vi "Anna_linescan2.0IngoHeucke.vi"() -> ()   [LabVIEW 2009]
panel:
  in  "Case Constant\n(See Context Help)":bool
  in  "Router":u32
  in  "save image to txt file":bool
  in  "threshold":cluster{"max":u32, "min":u32}
  in  "Header Path Ring":u16(ring)
  out "spots":i16
  in  "notes":string
  in  "new image":bool
  in  "exit":bool
  out "does a coinc image exist?":bool=TRUE
  in  "coincidence spot":bool
  in  "coincidence\nimage":bool
  out "LOADED HDR":bool
  out "Image LOADED":bool
  in  "settings":bool
  in  "Load Image":bool
  in  "F2-Image":bool
  in  "Lifetime pick":bool
  in  "Export":bool
  in  "TAC Window":bool
  in  "Spotfinder":bool
  in  "View FIFO Settings":bool
  in  "View Image Settings":bool
  in  "Load":bool
  out "total":i32
  out "gap":i32
  out "invalid":i32
  in  "plane":u32
  in  "router":u8(ring) items=["sum", "0", "1", "2", "3", "4", "5", "6"]
  in  "RGB or false color?":bool
  in  "16bit":bool
  out "already x spots":i16
  out "Int duplex?":bool
  out "16btimage?":bool
  out "Ampel":cluster{"RED":bool, "YELLOW":bool, "GREEN":bool}
  out "TACwinLoaded?":bool
  out "Boolean":bool
  in  "Image Path":path
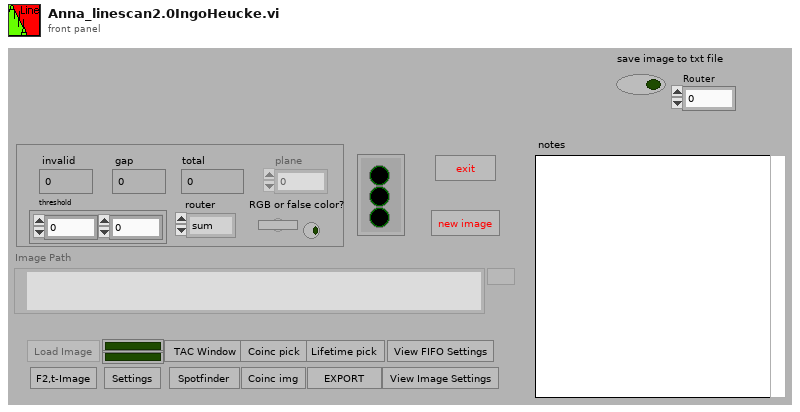
[diagram p1: front panel]
types:
  T1 = enum16{"Display", "change", "get", "save", "create text", "load", "Get Refnum"}
  T2 = enum16{"Get", "Set", "Change", "ini", "clear", "draw", "draw false"}
  T3 = enum16{"Ini", "Get", "Set", "Refresh", "dump", "move", "name"}
  T4 = enum16{"Ini", "Dump", "Colorpal", "Input", "Get"}
  T5 = enum16{"Display", "change", "Get", "Set", "Set Ken"}
  T6 = enum16{"Ini", "Get", "Set", "Draw", "Colorpal", "Dump", "Zoom"}
  T7 = cluster{"router":u8[], "macro times":dbl[], "micro times":u16[], "invalid":dbl[], "gap":dbl[]}
  T8 = typedef "Settings.ctl" = cluster{"threshold":cluster{"max":u32, "min":u32}, "RGB or false color":bool, "16bit":bool, "log/lin axis":u16, "spotsize button":bool, "Pixelsize":u16, "autoscale x":bool, "autoscale y":bool, "correlation":bool, "ADC-Resolution":i32, "F2-lifetime":cluster{"display tau":bool, "display F2":bool, "Palette Number lifetime":enum32{"Gray", "Binary", "Gradient", "Rainbow", "Temperature"}, "Palette Number F2":enum32{"Gray", "Binary", "Gradient", "Rainbow", "Temperature"}, "max tau-Value":dbl, "min tau-Value":dbl, "max F2-Value":dbl, "min F2-Value":dbl}, "TAC-Window 1":u16, "TAC-Window 2":u16, "false color palette":cluster{"1":u32, "2":u32, "3":u32, "4":u32, "5":u32, "6":u32, "7":u32, "8":u32, "8 2":u32, "8 3":u32, "8 4":u32, "8 5":u32}}
  T9 = enum32{"existing file", "new file", "new or existing file", "existing dir", "new dir", "new or existing dir", "existing file (use LLBs)", "new file (use LLBs)", "new or existing file (use LLBs)", "new or existing file or directory (use LLBs)"}
  T10 = typedef "ImageSettings.ctt" = cluster{"Start Position (µm)":cluster{"x":dbl, "y":dbl, "z":dbl}, "End Position (µm)":cluster{"x":dbl, "y":dbl, "z":dbl}, "Image Resolution (nm/pixel)":cluster{"x":dbl, "y":dbl, "z":dbl}, "Image Size (µm)":cluster{"x":dbl, "y":dbl, "z":dbl}, "Image Size (pixel)":cluster{"x":u32, "y":u32, "z":u32}, "Time Resolution\n(ms/pixel)":dbl, "1st Axis":u16, "2nd Axis":u16, "Retrace":bool, "Estimated Time":string}
  T11 = typedef "FIFOSettings_BH.ctt" = cluster{"Measurement":cluster{"Binning (ms)":sgl, "External Trigger Condition":u16, "Stop Condition:":u16, "Stop Count":dbl, "Buffer Size (Photons)":u16, "No of Channels":u16, "Ext Latch Delay":i16}, "ADC":cluster{"Module":u16, "ADC Resolution":i32, "Dither Range":i16, "Count Increment":i16, "Macro Time Clock":i16}, "SYNC":cluster{"SYNC ZC Level (mV)":sgl, "SYNC Freq Divider":i16, "SYNC Holdoff (ns)":sgl, "SYNC Threshold (mV)":sgl}, "TAC":cluster{"TAC Range (ns)":sgl, "TAC Gain":i16, "TAC Offset (%)":sgl, "TAC Limit Low (%)":sgl, "TAC Limit High (%)":sgl}, "CFD":cluster{"CFD Limit Low (mV)":sgl, "CFD Limit High (mV)":sgl, "CFD ZC Level (mV)":sgl, "CFD Holdoff (ns)":sgl}}
  T12 = typedef "spotproperties.ctl" = cluster{"draw?":bool, "plane":u32, "Coordinates":i32[], "TACWindow":cluster{"TACWindow1":i32, "TACWindow2":i32}, "Lifetime[ns]":ext[], "tauerror":dbl[], "F2-Value overall":dbl, "overall intensity":u32[], "F2-Value TAC":dbl, "TAC intensity":u32[], "Decay":u32[][]}
  T13 = enum16{"open", "replace", "create", "open or create", "replace or create", "replace or create with confirmation"}
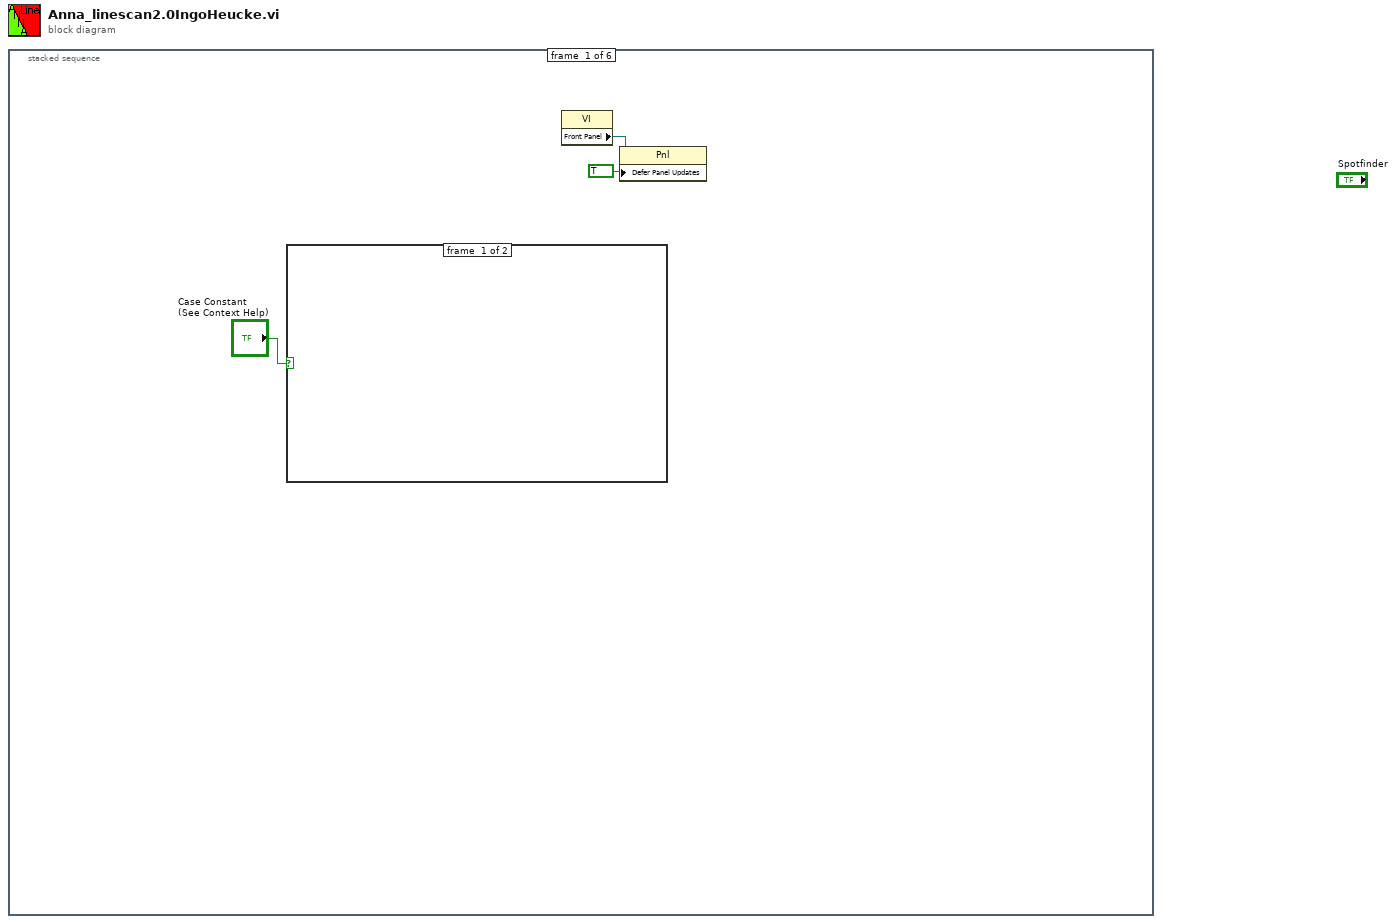
[diagram p0: block diagram]
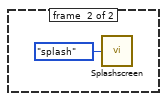
[diagram p2: hidden frame]
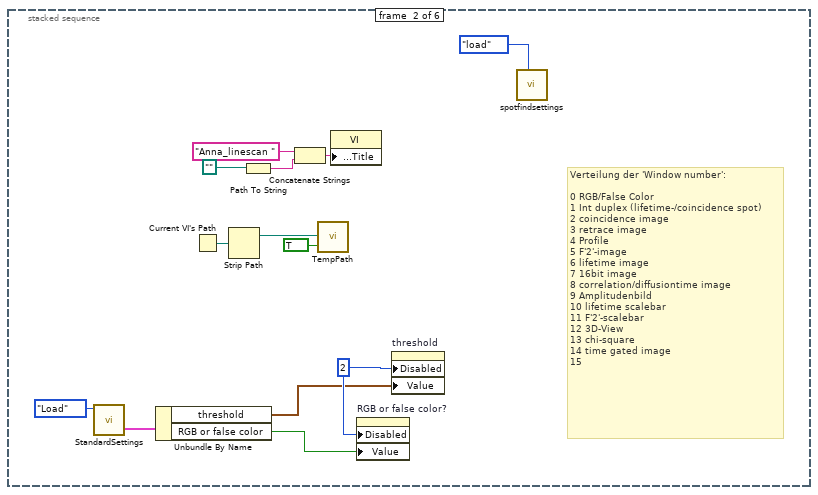
[diagram p3: hidden frame]
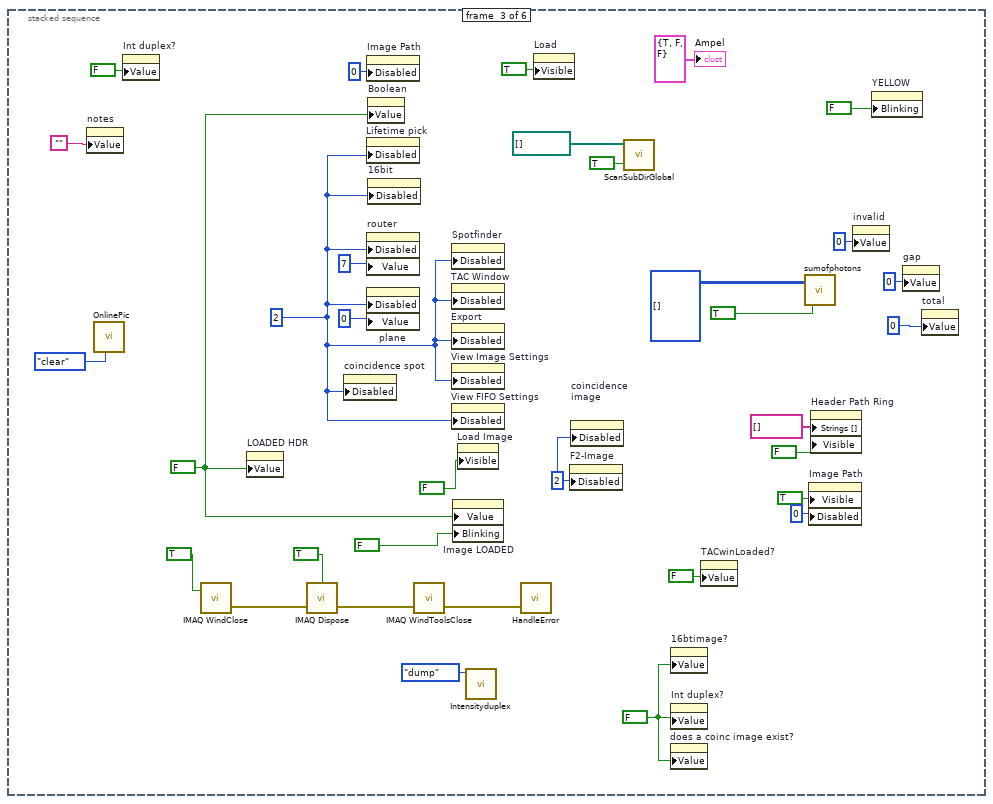
[diagram p4: hidden frame]
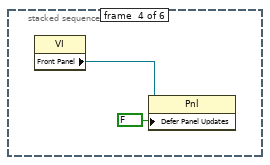
[diagram p5: hidden frame]
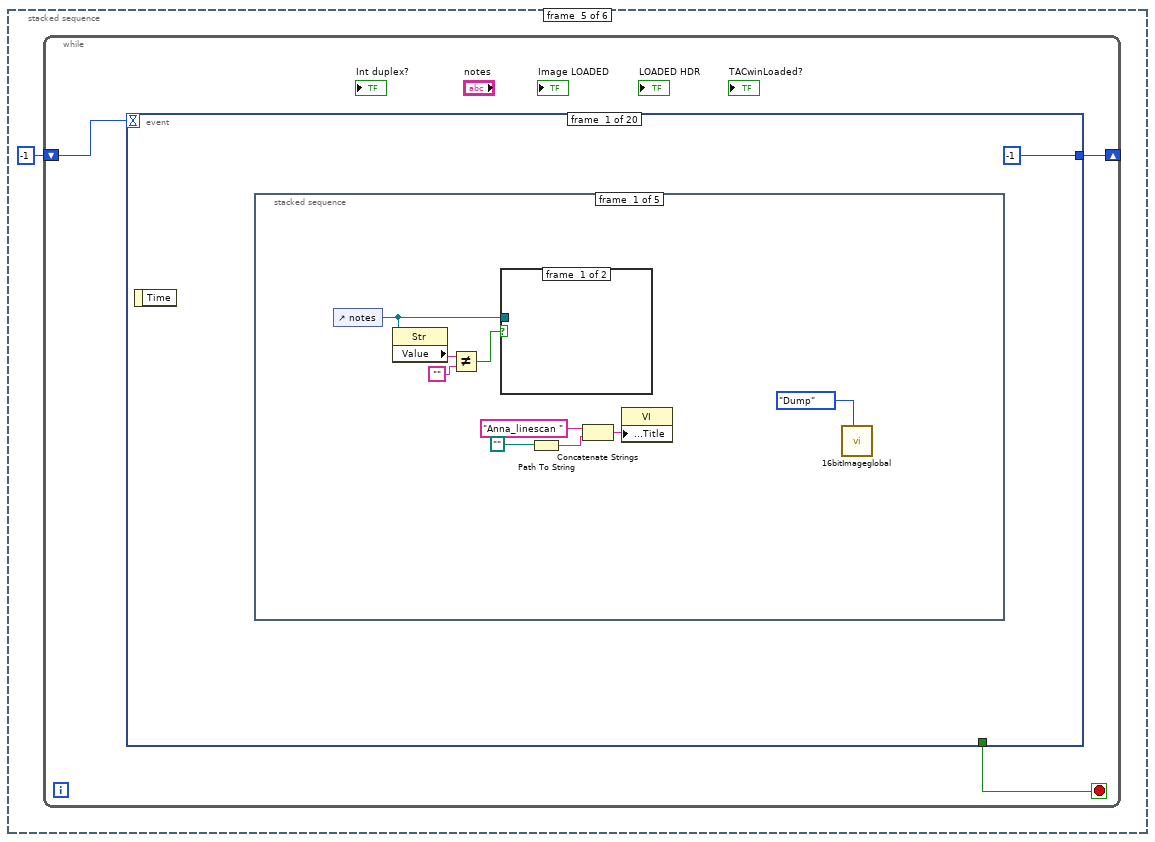
[diagram p6: hidden frame]
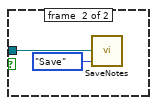
[diagram p7: hidden frame]
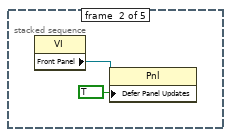
[diagram p8: hidden frame]
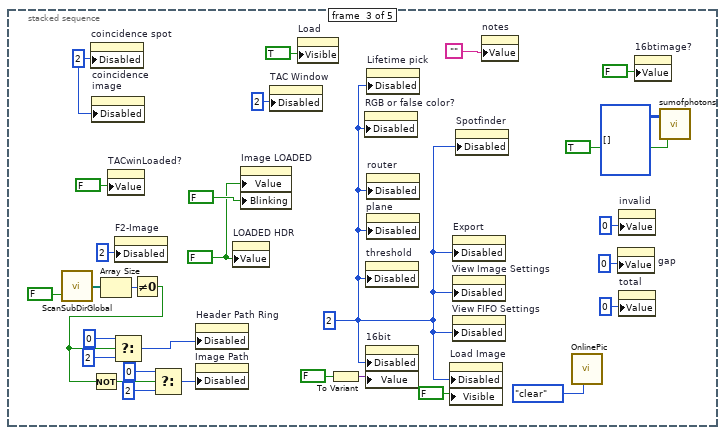
[diagram p9: hidden frame]
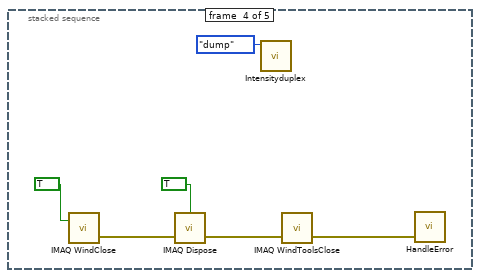
[diagram p10: hidden frame]
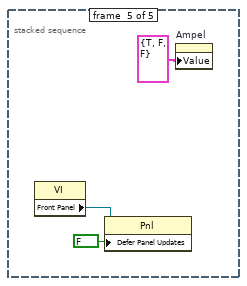
[diagram p11: hidden frame]
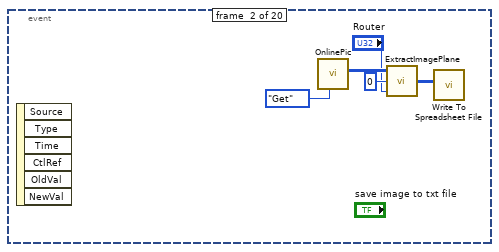
[diagram p12: hidden frame]
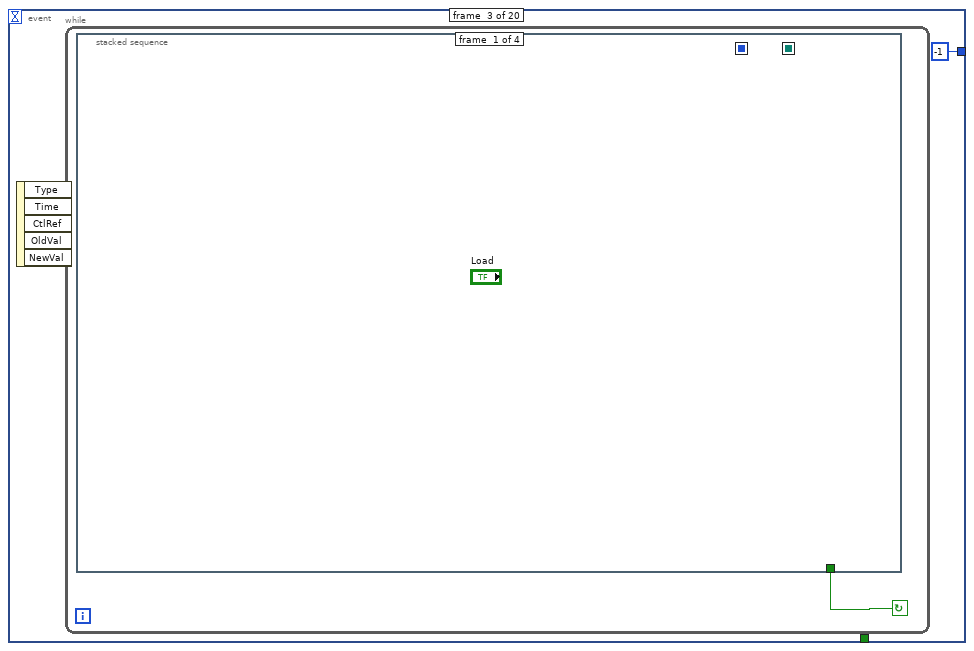
[diagram p13: hidden frame]
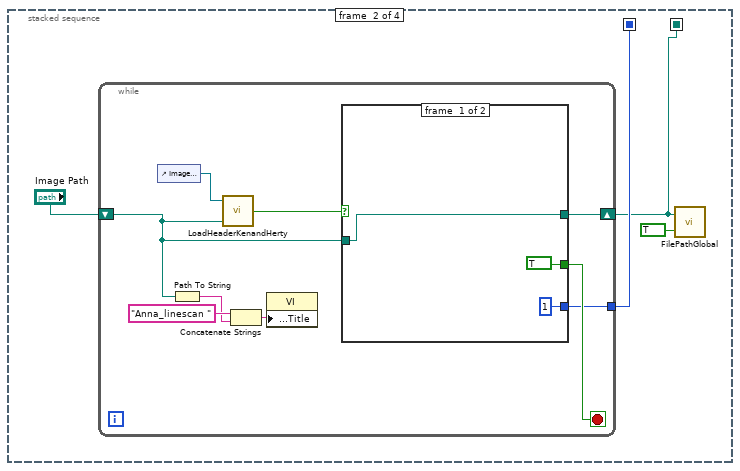
[diagram p14: hidden frame]
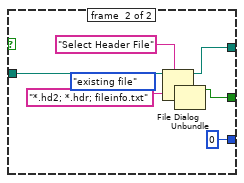
[diagram p15: hidden frame]
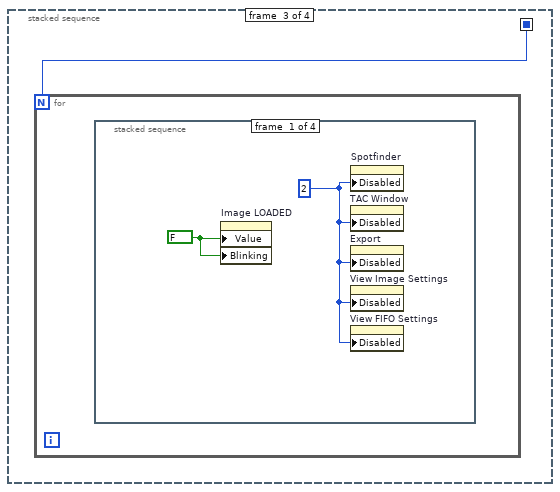
[diagram p16: hidden frame]
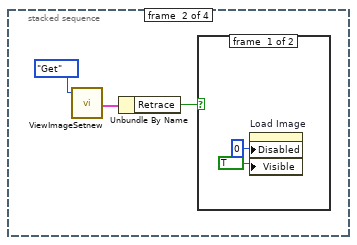
[diagram p17: hidden frame]
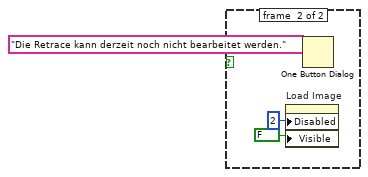
[diagram p18: hidden frame]
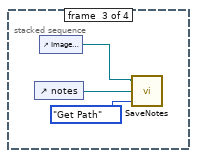
[diagram p19: hidden frame]
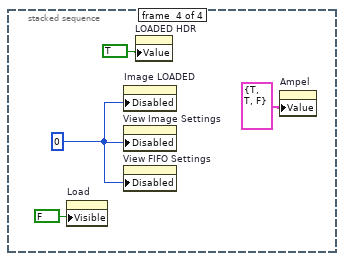
[diagram p20: hidden frame]
diagram:
  n1 = stacked-sequence {
    frame #0 {
      n2 = case shown="False" "Case Constant\n(See Context Help)" {
        frame #0 {
        }
        frame #1 {
          n3 = call "Splashscreen.vi"("Mode"=enum16{"splash", "dialog"}."splash") -> ()  [unwired: 1 in]
        }
      }
      n4 = property class="VI"() -> ("Front Panel"=w2:refnum<vi>)  [unwired: 2 in, 2 out]
      n5 = property class="Pnl"(reference=w2, "Defer Panel Updates"=TRUE) -> ()  [unwired: 1 in, 2 out]
    }
    frame #1 {
      w6 = u8 2 ("Disabled")
      # "Verteilung der 'Window number':\n\n0 RGB/False Color\n1 Int duplex (lifetime-/coincidence spot)\n2 coincidence image\n3 retrace image\n4 Profile\n5 F'2'-image\n6 lifetime image\n7 16bit image\n8 correlation/diffusiontime image\n9 Amplitudenbild\n10 lifetime scalebar\n11 F'2'-scalebar\n12 3D-View\n13 chi-square\n14 time gated image\n15"
      n6 = call "StandardSettings.vi"("Enum"=enum16{"Load", "get", "Save", "set"}."Load") -> ("StandardSettings"=w7:T8)  [unwired: 4 in]
      n7 = Unbundle By Name(w7) -> ("threshold"=w5:cluster{"max":u32, "min":u32}, "RGB or false color"=w8:bool)
      n8 = Current VI's Path() -> (path=w17:path)
      n9 = Strip Path(path=w17) -> (stripped path=w16:path)  [unwired: 1 out]
      n10 = Path To String(path=path "") -> (string=w12:string)
      n11 = Concatenate Strings("Anna_linescan " ("string"), w12) -> (w14:string)
      n12 = call "TempPath.vi"("change"=TRUE, "stripped path"=w16) -> ()  [unwired: 1 in, 1 out]
      n13 = property class="VI"("Front Panel Window:Title"=w14) -> ()  [unwired: 2 in, 2 out]
      n14 = property on="RGB or false color?" class="Boolean (strict)"("Disabled"=w6, "Value"=w8) -> ()  [unwired: 2 in, 2 out]
      n15 = property on="threshold" class="Clust (strict)"("Disabled"=w6, "Value"=w5) -> ()  [unwired: 2 in, 2 out]
      n16 = call "spotfindsettings.vi"("Enum"=T1."load") -> ()  [unwired: 8 in, 3 out]
    }
    frame #2 {
      w31 = FALSE
      w30 = u8 2 ("Disabled")
      w42 = FALSE ("Boolean")
      w20 = u8 2 ("Disabled")
      n17 = property on="notes" class="String"("Value"="") -> ()  [unwired: 2 in, 2 out]
      n18 = call "OnlinePic.vi"("action"=T2."clear" ("Enum")) -> ()  [unwired: 6 in, 5 out]
      n19 = property on="Int duplex?" class="Boolean (strict)"("Value"=FALSE ("Boolean 2")) -> ()  [unwired: 2 in, 2 out]
      n20 = call "IMAQ WindClose"("Close All Windows (False)"=TRUE ("Close All Windows (N)")) -> ("error out"=w47:errorcluster)  [unwired: 5 in]
      n21 = property on="LOADED HDR" class="Bool (strict)"("Value"=w42) -> ()  [unwired: 2 in, 2 out]
      n22 = call "IMAQ Dispose"("All Images? (No)"=TRUE, "error in (no error)"=w47) -> ("error out"=w48:errorcluster)  [unwired: 4 in]
      n23 = property on="coincidence spot" class="Boolean"("Disabled"=w20) -> ()  [unwired: 2 in, 2 out]
      n24 = property on="Image Path" class="Path"("Disabled"=u8 0) -> ()  [unwired: 2 in, 2 out]
      n25 = property on="Lifetime pick" class="Boolean"("Disabled"=w20) -> ()  [unwired: 2 in, 2 out]
      n26 = property on="router" class="Ring (strict)"("Disabled"=w20, "Value"=u8 7 ("router")) -> ()  [unwired: 2 in, 2 out]
      n27 = property on="plane" class="DigNum (strict)"("Disabled"=w20, "Value"=u32 0 ("plane")) -> ()  [unwired: 2 in, 2 out]
      n28 = property on="Boolean" class="Bool (strict)"("Value"=w42) -> ()  [unwired: 2 in, 2 out]
      n29 = property on="16bit" class="Boolean"("Disabled"=w20) -> ()  [unwired: 2 in, 2 out]
      n30 = call "IMAQ WindToolsClose"("error in (no error)"=w48) -> ("error out"=w46:errorcluster)  [unwired: 5 in]
      n31 = property on="Spotfinder" class="Boolean"("Disabled"=w20) -> ()  [unwired: 2 in, 2 out]
      n32 = property on="TAC Window" class="Boolean"("Disabled"=w20) -> ()  [unwired: 2 in, 2 out]
      n33 = property on="Export" class="Boolean"("Disabled"=w20) -> ()  [unwired: 2 in, 2 out]
      n34 = property on="View Image Settings" class="Boolean"("Disabled"=w20) -> ()  [unwired: 2 in, 2 out]
      n35 = property on="View FIFO Settings" class="Boolean"("Disabled"=w20) -> ()  [unwired: 2 in, 2 out]
      n36 = property on="Image LOADED" class="Boolean (strict)"("Value"=w42, "Blinking"=FALSE) -> ()  [unwired: 2 in, 2 out]
      n37 = property on="Load Image" class="Boolean"("Visible"=FALSE) -> ()  [unwired: 2 in, 2 out]
      n38 = call "Intensityduplex.vi"("Enum"=T3."dump") -> ()  [unwired: 4 in, 2 out]
      n39 = call "HandleError.vi"("error in (no error)"=w46) -> ()
      n40 = property on="Load" class="Bool"("Visible"=TRUE) -> ()  [unwired: 2 in, 2 out]
      n41 = property on="F2-Image" class="Boolean"("Disabled"=w30) -> ()  [unwired: 2 in, 2 out]
      n42 = property on="coincidence\nimage" class="Bool"("Disabled"=w30) -> ()  [unwired: 2 in, 2 out]
      n43 = call "ScanSubDirGlobal.vi"("set"=TRUE, "Array 2"=path[] []) -> ()  [unwired: 1 out]
      n44 = property on="16btimage?" class="Boolean (strict)"("Value"=w31) -> ()  [unwired: 2 in, 2 out]
      n45 = property on="Int duplex?" class="Boolean (strict)"("Value"=w31) -> ()  [unwired: 2 in, 2 out]
      n46 = property on="does a coinc image exist?" class="Boolean (strict)"("Value"=w31) -> ()  [unwired: 2 in, 2 out]
      n47 = property on="TACwinLoaded?" class="Boolean (strict)"("Value"=FALSE ("TACwinLoaded?")) -> ()  [unwired: 2 in, 2 out]
      n48 = call "sumofphotons.vi"("s"=TRUE, "sum of photons"=u32[][][][] []) -> ()  [unwired: 1 out]
      n49 = property on="Image Path" class="Path"("Visible"=TRUE, "Disabled"=u8 0) -> ()  [unwired: 2 in, 2 out]
      n50 = property on="Header Path Ring" class="Ring (strict)"("Strings []"=string[] [], "Visible"=FALSE) -> ()  [unwired: 2 in, 2 out]
      n51 = property on="invalid" class="DigNum (strict)"("Value"=u32 0 ("invalid photons")) -> ()  [unwired: 2 in, 2 out]
      n52 = property on="YELLOW" class="Boolean (strict)"("Blinking"=FALSE) -> ()  [unwired: 2 in, 2 out]
      n53 = property on="gap" class="DigNum (strict)"("Value"=u32 0 ("gap photons")) -> ()  [unwired: 2 in, 2 out]
      n54 = property on="total" class="DigNum (strict)"("Value"=u32 0 ("invalid photons")) -> ()  [unwired: 2 in, 2 out]
      "Ampel" <- cluster{"RED":bool, "YELLOW":bool, "GREEN":bool} {"RED"=TRUE, "YELLOW"=FALSE, "GREEN"=FALSE} ("Ampel")
    }
    frame #3 {
      n55 = property class="VI"() -> ("Front Panel"=w51:refnum<vi>)  [unwired: 2 in, 2 out]
      n56 = property class="Pnl"(reference=w51, "Defer Panel Updates"=FALSE) -> ()  [unwired: 1 in, 2 out]
    }
    frame #4 {
      n57 = while {
        shift-right: [w55] -> _
        shift-left: -1 -> [w54]
        stop <- w56 stop-if-true
        n58 = event shown="[2] \"Load\": Value Change" {
          selector: _ -> [_ _ _ _ _ _ _ _ _ _ _ _ _ _ _ _ _ _ _ _]
          dyn-events: _ -> [_ _ _ _ _ _ _ _ _ _ _ _ _ _ _ _ _ _ _ _]
          timeout: w54 -> [_ _ _ _ _ _ _ _ _ _ _ _ _ _ _ _ _ _ _ _]
          tunnel: [_ _ _ _ _ FALSE ("T button?") _ _ _ _ _ _ _ _ _ _ w463 _ TRUE w841] -> w56
          tunnel: [-1 _ -1 -1 -1 -1 100 -1 -1 -1 -1 -1 -1 -1 -1 -1 -1 -1 _ _] -> w55
          event #0 {
            n59 = event-data() -> ()  [unwired: 1 in, 1 out]
            n60 = stacked-sequence {
              frame #0 {
                n61 = control-ref of="notes"() -> (w66:refnum<vi>)
                n62 = property class="Str"(reference=w66) -> ("Value"=w59:string)  [unwired: 1 in, 2 out]
                n63 = Not Equal?(x=w59, y="") -> (x != y?=w58:bool)
                n64 = case shown="True" w58 {
                  tunnel: w66 -> [_ w67]
                  frame #0 {
                  }
                  frame #1 {
                    n65 = call "SaveNotes.vi"("Enum"=enum16{"Get Path", "Read", "Save"}."Save", "String"=w67) -> ()  [unwired: 3 in]
                  }
                }
                n66 = Path To String(path=path "") -> (string=w63:string)
                n67 = Concatenate Strings("Anna_linescan " ("string"), w63) -> (w65:string)
                n68 = property class="VI"("Front Panel Window:Title"=w65) -> ()  [unwired: 2 in, 2 out]
                n69 = call "16bitImageglobal.vi"("Enum"=T4."Dump") -> ()  [unwired: 4 in, 4 out]
              }
              frame #1 {
                n70 = property class="VI"() -> ("Front Panel"=w69:refnum<vi>)  [unwired: 2 in, 2 out]
                n71 = property class="Pnl"(reference=w69, "Defer Panel Updates"=TRUE) -> ()  [unwired: 1 in, 2 out]
              }
              frame #2 {
                w80 = u8 2 ("Disabled")
                w76 = FALSE ("Boolean")
                w71 = u8 2 ("Disabled")
                n72 = call "ScanSubDirGlobal.vi"("set"=FALSE) -> ("Array"=w89:path[])  [unwired: 1 in]
                n73 = property on="coincidence spot" class="Bool"("Disabled"=w80) -> ()  [unwired: 2 in, 2 out]
                n74 = property on="coincidence\nimage" class="Bool"("Disabled"=w80) -> ()  [unwired: 2 in, 2 out]
                n75 = Array Size(array=w89) -> (size(s)=w88:i32)
                n76 = property on="TACwinLoaded?" class="Boolean (strict)"("Value"=FALSE ("TACwinLoaded?")) -> ()  [unwired: 2 in, 2 out]
                n77 = property on="F2-Image" class="Boolean"("Disabled"=u8 2) -> ()  [unwired: 2 in, 2 out]
                n78 = Not Equal To 0?(x=w88) -> (x != 0?=w85:bool)
                n79 = Not(x=w85) -> (.not. x?=w84:bool)
                n80 = Select(t=u8 0 ("Disabled"), s=w85, f=u8 2 ("Disabled")) -> (s? t:f=w83:u8)
                n81 = Select(t=u8 0 ("Disabled"), s=w84, f=u8 2 ("Disabled")) -> (s? t:f=w82:u8)
                n82 = property on="Header Path Ring" class="Ring (strict)"("Disabled"=w83) -> ()  [unwired: 2 in, 2 out]
                n83 = property on="Image Path" class="Path"("Disabled"=w82) -> ()  [unwired: 2 in, 2 out]
                n84 = property on="LOADED HDR" class="Bool (strict)"("Value"=w76) -> ()  [unwired: 2 in, 2 out]
                n85 = property on="Image LOADED" class="Boolean (strict)"("Value"=w76, "Blinking"=FALSE) -> ()  [unwired: 2 in, 2 out]
                n86 = property on="TAC Window" class="Boolean"("Disabled"=2) -> ()  [unwired: 2 in, 2 out]
                n87 = property on="Load" class="Bool"("Visible"=TRUE) -> ()  [unwired: 2 in, 2 out]
                n88 = To Variant(anything=FALSE ("16btimage?")) -> (Variant=w73:variant)
                n89 = property on="RGB or false color?" class="Boolean (strict)"("Disabled"=w71) -> ()  [unwired: 2 in, 2 out]
                n90 = property on="threshold" class="Clust (strict)"("Disabled"=w71) -> ()  [unwired: 2 in, 2 out]
                n91 = property on="16bit" class="Boolean"("Disabled"=w71, "Value"=w73) -> ()  [unwired: 2 in, 2 out]
                n92 = property on="Lifetime pick" class="Boolean"("Disabled"=w71) -> ()  [unwired: 2 in, 2 out]
                n93 = property on="router" class="Ring (strict)"("Disabled"=w71) -> ()  [unwired: 2 in, 2 out]
                n94 = property on="plane" class="DigNum (strict)"("Disabled"=w71) -> ()  [unwired: 2 in, 2 out]
                n95 = property on="Load Image" class="Boolean"("Disabled"=w71, "Visible"=FALSE) -> ()  [unwired: 2 in, 2 out]
                n96 = property on="Export" class="Boolean"("Disabled"=w71) -> ()  [unwired: 2 in, 2 out]
                n97 = property on="View Image Settings" class="Boolean"("Disabled"=w71) -> ()  [unwired: 2 in, 2 out]
                n98 = property on="View FIFO Settings" class="Boolean"("Disabled"=w71) -> ()  [unwired: 2 in, 2 out]
                n99 = property on="Spotfinder" class="Boolean"("Disabled"=w71) -> ()  [unwired: 2 in, 2 out]
                n100 = property on="notes" class="String"("Value"="") -> ()  [unwired: 2 in, 2 out]
                n101 = call "OnlinePic.vi"("action"=T2."clear" ("Enum")) -> ()  [unwired: 6 in, 5 out]
                n102 = property on="gap" class="DigNum (strict)"("Value"=u32 0 ("gap photons")) -> ()  [unwired: 2 in, 2 out]
                n103 = property on="invalid" class="DigNum (strict)"("Value"=u32 0 ("invalid photons")) -> ()  [unwired: 2 in, 2 out]
                n104 = property on="total" class="DigNum (strict)"("Value"=u32 0 ("invalid photons")) -> ()  [unwired: 2 in, 2 out]
                n105 = property on="16btimage?" class="Boolean (strict)"("Value"=FALSE ("16btimage?")) -> ()  [unwired: 2 in, 2 out]
                n106 = call "sumofphotons.vi"("s"=TRUE, "sum of photons"=u32[][][][] []) -> ()  [unwired: 1 out]
              }
              frame #3 {
                n107 = call "IMAQ WindClose"("Close All Windows (False)"=TRUE ("Close All Windows (N)")) -> ("error out"=w104:errorcluster)  [unwired: 5 in]
                n108 = call "IMAQ Dispose"("All Images? (No)"=TRUE, "error in (no error)"=w104) -> ("error out"=w105:errorcluster)  [unwired: 4 in]
                n109 = call "Intensityduplex.vi"("Enum"=T3."dump") -> ()  [unwired: 4 in, 2 out]
                n110 = call "IMAQ WindToolsClose"("error in (no error)"=w105) -> ("error out"=w101:errorcluster)  [unwired: 5 in]
                n111 = call "HandleError.vi"("error in (no error)"=w101) -> ()
              }
              frame #4 {
                n112 = property class="VI"() -> ("Front Panel"=w107:refnum<vi>)  [unwired: 2 in, 2 out]
                n113 = property class="Pnl"(reference=w107, "Defer Panel Updates"=FALSE) -> ()  [unwired: 1 in, 2 out]
                n114 = property on="Ampel" class="Clust (strict)"("Value"=cluster{"RED":bool, "RED 2":bool, "RED 3":bool} {"RED"=TRUE, "RED 2"=FALSE, "RED 3"=FALSE} ("Ampel")) -> ()  [unwired: 2 in, 2 out]
              }
            }
          }
          event #1 {
            n115 = event-data() -> ()  [unwired: 1 in, 6 out]
            n116 = call "OnlinePic.vi"("action"=enum16{"Get", "Set", "Change", "ini"}."Get" ("Enum")) -> ("Sum of Photons"=w113:u32[][][][])  [unwired: 6 in, 4 out]
            n117 = call "ExtractImagePlane.vi"("Router"="Router", "Plane"=u32 0, "Trace"=w113) -> ("Intensity"=w110:u32[][])
            n118 = call "Write To Spreadsheet File.vi"("2D data"=w110) -> ()  [unwired: 7 in, 1 out]
          }
          event #2 {
            n119 = event-data() -> ()  [unwired: 1 in, 5 out]
            n120 = while {
              stop <- w116 continue-if-true
              n121 = stacked-sequence {
                seq-local: [_ w119 _ _] -> [_ _ w140 _]
                seq-local: [_ w117 _ _] -> [_ _ _ w159]
                tunnel: [_ _ _ w158] -> w116
                frame #0 {
                }
                frame #1 {
                  n122 = while {
                    shift-right: [w122] -> w117
                    shift-left: "Image Path" -> [w123]
                    tunnel: [w121] -> w119
                    stop <- w124 stop-if-true
                    n123 = control-ref of="Image Path"() -> (w129:refnum<vi>)
                    n124 = Path To String(path=w123) -> (string=w126:string)
                    n125 = call "LoadHeaderKenandHerty.vi"("appended path"=w123, "reference"=w129) -> ("unsuccesful?"=w125:bool)  [unwired: 3 in]
                    n126 = Concatenate Strings("Anna_linescan " ("string"), w126) -> (w128:string)
                    n127 = property class="VI"("Front Panel Window:Title"=w128) -> ()  [unwired: 2 in, 2 out]
                    n128 = case shown="False" w125 {
                      tunnel: w123 -> [w130 w139]
                      tunnel: [TRUE w135] -> w124
                      tunnel: [w130 w137] -> w122
                      tunnel: [1 0] -> w121
                      frame #0 {
                      }
                      frame #1 {
                        (unwired) T9."existing file" ("select mode (2)")
                        n129 = File Dialog(6:"*.hd2; *.hdr; fileinfo.txt" ("pattern"), 7:"Select Header File" ("prompt"), 11:w139) -> (0:w133:errorcluster, 1:w135:bool, 3:w137:path)  [unwired: 4 in, 1 out]
                        n130 = Unbundle(w133) -> ()  [unwired: 3 out]
                      }
                    }
                  }
                  n131 = call "FilePathGlobal.vi"("Image Path"=w117, "set?"=TRUE) -> ()  [unwired: 3 out]
                }
                frame #2 {
                  n132 = for {
                    N: w140 -> [_]
                    n133 = stacked-sequence {
                      frame #0 {
                        w142 = u8 2 ("Disabled")
                        w141 = FALSE ("Boolean")
                        n134 = property on="Image LOADED" class="Boolean (strict)"("Value"=w141, "Blinking"=w141) -> ()  [unwired: 2 in, 2 out]
                        n135 = property on="Spotfinder" class="Boolean"("Disabled"=w142) -> ()  [unwired: 2 in, 2 out]
                        n136 = property on="TAC Window" class="Boolean"("Disabled"=w142) -> ()  [unwired: 2 in, 2 out]
                        n137 = property on="Export" class="Boolean"("Disabled"=w142) -> ()  [unwired: 2 in, 2 out]
                        n138 = property on="View Image Settings" class="Boolean"("Disabled"=w142) -> ()  [unwired: 2 in, 2 out]
                        n139 = property on="View FIFO Settings" class="Boolean"("Disabled"=w142) -> ()  [unwired: 2 in, 2 out]
                      }
                      frame #1 {
                        n140 = call "ViewImageSetnew.vi"("action"=enum16{"Display", "change", "Get", "Set"}."Get" ("Enum")) -> ("Image Settings"=w144:T10)  [unwired: 2 in]
                        n141 = Unbundle By Name(w144) -> ("Retrace"=w143:bool)
                        n142 = case shown="False" w143 {
                          frame #0 {
                            n143 = property on="Load Image" class="Boolean"("Disabled"=u8 0, "Visible"=TRUE) -> ()  [unwired: 2 in, 2 out]
                          }
                          frame #1 {
                            n144 = property on="Load Image" class="Boolean"("Disabled"=u8 2, "Visible"=FALSE) -> ()  [unwired: 2 in, 2 out]
                            n145 = One Button Dialog(message="Die Retrace kann derzeit noch nicht bearbeitet werden.") -> ()  [unwired: 1 in, 1 out]
                          }
                        }
                      }
                      frame #2 {
                        n146 = control-ref of="notes"() -> (w153:refnum<vi>)
                        n147 = control-ref of="Image Path"() -> (w151:refnum<vi>)
                        n148 = call "SaveNotes.vi"("Enum"=enum16{"Get Path", "Read", "Save"}."Get Path", "String"=w153, "Path"=w151) -> ()  [unwired: 2 in]
                      }
                      frame #3 {
                        w156 = u8 0 ("Disabled")
                        n149 = property on="Load" class="Bool"("Visible"=FALSE) -> ()  [unwired: 2 in, 2 out]
                        n150 = property on="Image LOADED" class="Boolean (strict)"("Disabled"=w156) -> ()  [unwired: 2 in, 2 out]
                        n151 = property on="View Image Settings" class="Boolean"("Disabled"=w156) -> ()  [unwired: 2 in, 2 out]
                        n152 = property on="View FIFO Settings" class="Boolean"("Disabled"=w156) -> ()  [unwired: 2 in, 2 out]
                        n153 = property on="LOADED HDR" class="Bool (strict)"("Value"=TRUE ("Boolean")) -> ()  [unwired: 2 in, 2 out]
                        n154 = property on="Ampel" class="Clust (strict)"("Value"=cluster{"RED":bool, "RED 2":bool, "RED 3":bool} {"RED"=TRUE, "RED 2"=TRUE, "RED 3"=FALSE} ("Ampel")) -> ()  [unwired: 2 in, 2 out]
                      }
                    }
                  }
                }
                frame #3 {
                  n155 = stacked-sequence {
                    tunnel: [_ _ _ _ _ _ _ _ _ _ _ w241] -> _
                    tunnel: w159 -> [_ _ _ _ _ _ _ _ _ _ _ w241]
                    tunnel: [_ _ _ _ _ _ _ _ _ _ _ w228] -> w158
                    frame #0 {
                      n156 = property on="Image LOADED" class="Boolean (strict)"("Blinking"=TRUE) -> ()  [unwired: 2 in, 2 out]
                      n157 = property on="Image Path" class="Path"("Disabled"=u8 2) -> ()  [unwired: 2 in, 2 out]
                      n158 = property on="Load Image" class="Boolean"("Disabled"=u8 2) -> ()  [unwired: 2 in, 2 out]
                      n159 = call "sumofphotons.vi"("s"=TRUE, "sum of photons"=u32[][][][] []) -> ()  [unwired: 1 out]
                    }
                    frame #1 {
                      n160 = call "WriteTempData.vi"("Enum"=enum16{"create new", "write", "close"}."create new") -> ("error out"=w165:errorcluster)  [unwired: 4 in, 1 out]
                      n161 = call "HandleError.vi"("error in (no error)"=w165) -> ()
                    }
                    frame #2 {
                      n162 = call "fileformatGlobal.vi"("changed"=FALSE) -> ("fileformat out"=w167:enum16{"Herty", "Ken", "SPC130", "HydraHarp"})  [unwired: 1 in]
                      n163 = control-ref of="Image Path"() -> (w169:refnum<vi>)
                      n164 = case shown="\"HydraHarp\"" w167 {
                        tunnel: w169 -> [w170 w171 w172 w173]
                        frame #0 {
                          n165 = call "LoadData.vi"("Path"=w170) -> ()  [unwired: 2 in, 3 out]
                        }
                        frame #1 {
                          n166 = call "LoadDataSPC130.vi"("Path"=w171) -> ()  [unwired: 2 in, 3 out]
                        }
                        frame #2 {
                          n167 = call "LoadDataHH.vi"("Path"=w172) -> ()  [unwired: 2 in, 3 out]
                        }
                        frame #3 {
                          n168 = call "LoadDataKen.vi"("Path"=w173) -> ()  [unwired: 5 in]
                        }
                      }
                    }
                    frame #3 {
                      n169 = call "WriteTempData.vi"("Enum"=enum16{"create new", "write", "close"}."close") -> ("error out"=w174:errorcluster)  [unwired: 4 in, 1 out]
                      n170 = call "HandleError.vi"("error in (no error)"=w174) -> ()
                    }
                    frame #4 {
                      n171 = call "TotalRecall_Reload.vi"() -> ("gap"=→"gap":i32, "invalid"=→"invalid":i32, "valid"=→"total":i32)  [unwired: 4 in, 1 out]
                    }
                    frame #5 {
                      n172 = call "ViewFIFOSet.vi"("Enum"=T5."Get") -> ("FIFO Settings (Array)"=w185:T11[])  [unwired: 1 in]
                      n173 = Index Array(array=w185) -> (element=w186:T11)  [unwired: 1 in]
                      n174 = Array Size(array=w185) -> (size(s)=w181:i32)
                      n175 = Unbundle By Name(w186) -> ("Measurement.No of Channels"=w180:u16)
                      n176 = Multiply(x=w180, y=w181) -> (x*y=w179:i32)
                      n177 = for {
                        N: w179 -> [_]
                        tunnel: [w195] -> w184 mode=indexing
                        i -> [w196]
                        n178 = Number To Decimal String(number=w196) -> (decimal integer string=w195:string)  [unwired: 1 in]
                      }
                      n179 = Build Array (concatenate)("sum", w184) -> (w182:string[])
                      n180 = property on="router" class="Ring (strict)"("Strings []"=w182) -> ("Value"=w191:u8)  [unwired: 2 in, 2 out]
                      n181 = property on="plane" class="DigNum (strict)"() -> ("Value"=w192:u32)  [unwired: 2 in, 2 out]
                      n182 = property on="threshold" class="Clust (strict)"() -> ("Value"=w188:cluster{"max":u32, "min":u32})  [unwired: 2 in, 2 out]
                      n183 = call "sumofphotons.vi"("s"=FALSE) -> ("sum of photons out"=w189:u32[][][][])  [unwired: 1 in]
                      n184 = property on="RGB or false color?" class="Bool (strict)"() -> ("Value"=w193:bool)  [unwired: 2 in, 2 out]
                      n185 = call "OnlinePic.vi"("action"=T2."ini" ("Enum"), "RGB/False"=w193, "Threshold (max)"=w188, "plane"=w192, "router channel"=w191, "Array"=w189) -> ()  [unwired: 1 in, 5 out]
                    }
                    frame #6 {
                      n186 = call "ViewImageSetnew.vi"("action"=enum16{"Display", "change", "Get", "Set"}."Get" ("Enum")) -> ("Image Settings"=w198:T10)  [unwired: 2 in]
                      n187 = Unbundle By Name(w198) -> ("Image Size (pixel).z"=w199:u32)
                      n188 = case shown="0" w199 {
                        tunnel: [i8 2 w204] -> w200
                        tunnel: [u8 0 w204] -> w201
                        frame #0 {
                        }
                        frame #1 {
                          w204 = u8 0
                        }
                      }
                      n189 = property on="plane" class="DigNum (strict)"("Disabled"=w200, "Value"=w201) -> ()  [unwired: 2 in, 2 out]
                    }
                    frame #7 {
                      w205 = u8 0
                      n190 = property on="Image LOADED" class="Boolean (strict)"("Blinking"=FALSE, "Value"=TRUE ("Image LOADED")) -> ()  [unwired: 2 in, 2 out]
                      n191 = property on="Lifetime pick" class="Boolean"("Disabled"=w205) -> ()  [unwired: 2 in, 2 out]
                      n192 = property on="RGB or false color?" class="Boolean (strict)"("Disabled"=w205) -> ()  [unwired: 2 in, 2 out]
                      n193 = property on="16bit" class="Boolean"("Disabled"=w205) -> ()  [unwired: 2 in, 2 out]
                      n194 = property on="threshold" class="Clust (strict)"("Disabled"=w205) -> ()  [unwired: 2 in, 2 out]
                      n195 = property on="Spotfinder" class="Boolean"("Disabled"=w205) -> ()  [unwired: 2 in, 2 out]
                      n196 = property on="router" class="Ring (strict)"("Disabled"=w205) -> ()  [unwired: 2 in, 2 out]
                      n197 = property on="coincidence spot" class="Boolean"("Disabled"=w205) -> ()  [unwired: 2 in, 2 out]
                      n198 = property on="TAC Window" class="Boolean"("Disabled"=w205) -> ()  [unwired: 2 in, 2 out]
                      n199 = property on="Export" class="Bool"("Disabled"=w205) -> ()  [unwired: 2 in, 2 out]
                      n200 = property on="F2-Image" class="Boolean"("Disabled"=u8 0) -> ()  [unwired: 2 in, 2 out]
                      n201 = property on="coincidence\nimage" class="Bool"("Disabled"=w205) -> ()  [unwired: 2 in, 2 out]
                    }
                    frame #8 {
                      n202 = property on="Ampel" class="Clust (strict)"("Value"=cluster{"RED":bool, "RED 2":bool, "RED 3":bool} {"RED"=FALSE, "RED 2"=FALSE, "RED 3"=TRUE} ("Ampel")) -> ()  [unwired: 2 in, 2 out]
                    }
                    frame #9 {
                      n203 = stacked-sequence {
                        frame #0 {
                          n204 = property on="Ampel" class="Clust (strict)"("Value"=cluster{"RED":bool, "YELLOW":bool, "GREEN":bool} {"RED"=FALSE, "YELLOW"=FALSE, "GREEN"=FALSE} ("Ampel")) -> ("Controls[]"=w213:refnum<vi>[])  [unwired: 2 in, 2 out]
                          n205 = Index Array(array=w213, index=1) -> (element=w211:refnum<vi>)
                          n206 = property class="Ctl"(reference=w211, "Blinking"=TRUE) -> ()  [unwired: 1 in, 2 out]
                        }
                        frame #1 {
                          n207 = control-ref of="plane"() -> (w218:refnum<vi>)
                          n208 = control-ref of="TACwinLoaded?"() -> (w220:refnum<vi>)
                          n209 = control-ref of="16btimage?"() -> (w219:refnum<vi>)
                          n210 = control-ref of="router"() -> (w217:refnum<vi>)
                          n211 = control-ref of="Image Path"() -> (w221:refnum<vi>)
                          n212 = control-ref of="notes"() -> (w216:refnum<vi>)
                          n213 = control-ref of="Int duplex?"() -> (w222:refnum<vi>)
                          n214 = call "SpotFinderIngoHeucke.vi"("auto"=FALSE, "Int duplex?"=w222, "notes"=w216, "router 3"=w217, "plane 2"=w218, "Image Path"=w221, "16bit?"=w219, "TACwinLoaded?"=w220) -> ()  [unwired: 3 in]
                        }
                        frame #2 {
                          n215 = property on="Ampel" class="Clust (strict)"("Value"=cluster{"RED":bool, "YELLOW":bool, "GREEN":bool} {"RED"=FALSE, "YELLOW"=FALSE, "GREEN"=TRUE} ("Ampel")) -> ("Controls[]"=w226:refnum<vi>[])  [unwired: 2 in, 2 out]
                          n216 = Index Array(array=w226, index=1) -> (element=w224:refnum<vi>)
                          n217 = property class="Ctl"(reference=w224, "Blinking"=FALSE) -> ()  [unwired: 1 in, 2 out]
                        }
                      }
                    }
                    frame #10 {
                    }
                    frame #11 {
                      # "next file"
                      n218 = Strip Path(path=w241) -> (stripped path=w240:path, name=w237:string)
                      n219 = Strip Path(path=w240) -> (stripped path=w234:path, name=w236:string)
                      n220 = Scan From String(format string="%d", input string=w236) -> (output 1=w238:i32)  [unwired: 3 in, 3 out]
                      n221 = Increment(x=w238) -> (x+1=w235:i32)
                      n222 = Number To Decimal String(number=w235) -> (decimal integer string=w233:string)  [unwired: 1 in]
                      n223 = Search and Replace String(input string=w237, search string=w236, replace string=w233) -> (result string=w231:string)  [unwired: 5 in, 3 out]
                      n224 = Build Path(base path=w234, name or relative path=w233) -> (appended path=w232:path)
                      n225 = Build Path(base path=w232, name or relative path=w231) -> (appended path=w229:path)
                      n226 = call <vilib>:"Check if File or Folder Exists.vi"("path"=w229) -> ("file or folder exists?"=w228:bool)  [unwired: 8 in, 2 out]
                      n227 = call "FilePathGlobal.vi"("Image Path"=w229, "set?"=TRUE) -> ()  [unwired: 3 out]
                      n228 = local write "Image Path"(w229) -> ()
                    }
                  }
                }
              }
            }
          }
          event #3 {
            n229 = event-data() -> ()  [unwired: 1 in, 5 out]
          }
          event #4 {
            n230 = event-data() -> ()  [unwired: 1 in, 5 out]
            n231 = Unbundle By Name("threshold") -> ("max"=w248:u32, "min"=w247:u32)
            n232 = call "CheckPlane.vi"("plane 2"="plane") -> ("plane"=w249:u32)
            n233 = Max & Min(x=w248, y=w247) -> (max(x,y)=w246:u32, min(x,y)=w245:u32)
            n234 = Bundle By Name(cluster="threshold", "max"=w246, "min"=w245) -> (w243:cluster{"max":u32, "min":u32})
            n235 = property on="threshold" class="Cluster (strict)"("Value"=w243) -> ()  [unwired: 2 in, 2 out]
            n236 = property on="plane" class="DigNum (strict)"("Value"=w249) -> ()  [unwired: 2 in, 2 out]
            n237 = property on="16btimage?" class="Bool (strict)"() -> ("Value"=w258:bool)  [unwired: 2 in, 2 out]
            n238 = call "OnlinePic.vi"("action"=T2."Change" ("Enum"), "RGB/False"="RGB or false color?", "Threshold (max)"=w243, "plane"=w249, "router channel"="router") -> ()  [unwired: 2 in, 5 out]
            n239 = call "StandardSettings.vi"("Enum"=enum16{"Load", "get", "Save", "set"}."get") -> ("StandardSettings"=w254:T8)  [unwired: 4 in]
            n240 = Bundle By Name(cluster=w254, "threshold"=w243, "RGB or false color"="RGB or false color?") -> (w253:T8)
            n241 = case shown="True" w258 {
              tunnel: "router" -> [_ w263]
              tunnel: w249 -> [_ w262]
              frame #0 {
              }
              frame #1 {
                n242 = call "16bitImageglobal.vi"("Enum"=T4."Input", "plane"=w262, "router"=w263) -> ("error out"=w260:errorcluster)  [unwired: 2 in, 3 out]
                n243 = call "HandleError.vi"("error in (no error)"=w260) -> ()
              }
            }
            n244 = call "StandardSettings.vi"("StandardSettings"=w253, "Enum"=enum16{"Load", "get", "Save", "set"}."set") -> ()  [unwired: 3 in, 1 out]
          }
          event #5 {
            n245 = event-data() -> ()  [unwired: 1 in, 5 out]
            n246 = stacked-sequence {
              seq-local: [_ _ _ w294 _] -> [_ _ _ _ w299]
              frame #0 {
                n247 = property on="Ampel" class="Clust (strict)"("Value"=cluster{"RED":bool, "RED 2":bool, "RED 3":bool} {"RED"=FALSE, "RED 2"=FALSE, "RED 3"=FALSE} ("Ampel")) -> ()  [unwired: 2 in, 2 out]
                n248 = property on="TACwinLoaded?" class="Boolean (strict)"() -> ("Value"=w269:bool)  [unwired: 2 in, 2 out]
                n249 = call "Intensityduplex.vi"("Enum"=T3."dump") -> ()  [unwired: 4 in, 2 out]
                n250 = case shown="False" w269 {
                  frame #0 {
                    n251 = call "GetTACWindow.vi"("Enum"=enum16{"ini", "get", "quick"}."quick") -> ()  [unwired: 1 in, 9 out]
                  }
                  frame #1 {
                  }
                }
                n252 = property on="YELLOW" class="Boolean (strict)"("Blinking"=TRUE) -> ()  [unwired: 2 in, 2 out]
              }
              frame #1 {
                n253 = property on="threshold" class="Clust (strict)"() -> ("Value"=w271:cluster{"max":u32, "min":u32})  [unwired: 2 in, 2 out]
                n254 = call "StandardSettings.vi"("Enum"=enum16{"Load", "get", "Save", "set"}."get") -> ("StandardSettings"=w273:T8)  [unwired: 4 in]
                n255 = Bundle By Name(cluster=w273, "threshold"=w271) -> (w272:T8)
                n256 = property on="notes" class="String"() -> ("Value"=w277:string)  [unwired: 2 in, 2 out]
                n257 = Concatenate Strings(w277, "\n- lifetime picking" ("string")) -> (w276:string)
                n258 = call "StandardSettings.vi"("StandardSettings"=w272, "Enum"=enum16{"Load", "get", "Save", "set"}."set") -> ()  [unwired: 3 in, 1 out]
                n259 = control-ref of="Image Path"() -> (w281:refnum<vi>)
                n260 = property on="notes" class="String"("Value"=w276) -> ()  [unwired: 2 in, 2 out]
                n261 = call "WriteStoreData.vi"("Enum"=enum16{"Save", "Control"}."Control", "Image Path"=w281) -> ("already x spots"=→"already x spots":i16)  [unwired: 1 in]
              }
              frame #2 {
                n262 = property on="already x spots" class="Digital (strict)"() -> ("Value"=w284:i16)  [unwired: 2 in, 2 out]
                n263 = control-ref of="notes"() -> (w283:refnum<vi>)
                n264 = call "LifetimePickTACCube.vi"("notes 2"=w283, "already x spots"=w284) -> ("spots"=→"spots":i16)  [unwired: 1 in]
              }
              frame #3 {
                w293 = "%02d to %02d" ("format string")
                n265 = property on="already x spots" class="Digital (strict)"() -> ("Value"=w292:i16)  [unwired: 2 in, 2 out]
                n266 = property on="spots" class="Digital (strict)"() -> ("Value"=w291:i16)  [unwired: 2 in, 2 out]
                n267 = Greater?(x=w292, y=w291) -> (0:w290:bool)
                n268 = Decrement(x=w291) -> (x-1=w295:i16)
                n269 = Format Into String(format string=w293, initial string=" spots ", w292, w295) -> ()  [unwired: 1 in, 2 out]
                n270 = Format Into String(format string=w293, w292, w295) -> (resulting string=w294:string)  [unwired: 2 in, 1 out]
                n271 = Select(t=w293, s=w290, f="") -> (s? t:f=w288:string)
                n272 = call "Intensityduplex.vi"("Enum"=T3."name", "add string"=w288) -> ()  [unwired: 3 in, 2 out]
                n273 = call "OnlinePic.vi"("action"=T2."Get" ("Enum")) -> ("RGB/False out"=w286:bool, "Threshold (max) OUT"=w285:cluster{"max":u32, "min":u32})  [unwired: 6 in, 3 out]
                n274 = property on="RGB or false color?" class="Bool (strict)"("Value"=w286) -> ()  [unwired: 2 in, 2 out]
                n275 = property on="threshold" class="Clust (strict)"("Value"=w285) -> ()  [unwired: 2 in, 2 out]
              }
              frame #4 {
                n276 = call "StoreDatafromLifetimePick.vi"("Enum"=enum16{"clear", "Get", "Set", "Add"}."Get") -> ("Spots"=w298:T12[], "store s.th.?"=w303:bool)  [unwired: 1 in]
                n277 = case shown="True" w303 {
                  tunnel: w299 -> [_ w306]
                  tunnel: w298 -> [_ w305]
                  frame #0 {
                  }
                  frame #1 {
                    n278 = stacked-sequence {
                      tunnel: w306 -> [_ w311]
                      tunnel: w305 -> [w307 _]
                      frame #0 {
                        n279 = control-ref of="Image Path"() -> (w309:refnum<vi>)
                        n280 = call "WriteStoreData.vi"("Spots"=w307, "Enum"=enum16{"Save", "Control"}."Save", "Image Path"=w309) -> ()  [unwired: 1 out]
                      }
                      frame #1 {
                        n281 = property on="notes" class="String"() -> ("Value"=w313:string)  [unwired: 2 in, 2 out]
                        n282 = Concatenate Strings(w313, "\npick result spots (" ("string"), w311, ") and decays stored in IMAGE PATH\n" ("string")) -> (w312:string)
                        n283 = property on="notes" class="String"("Value"=w312) -> ()  [unwired: 2 in, 2 out]
                      }
                    }
                  }
                }
                n284 = property on="Int duplex?" class="Boolean (strict)"("Value"=TRUE ("Boolean 2")) -> ()  [unwired: 2 in, 2 out]
                n285 = property on="Ampel" class="Clust (strict)"("Value"=cluster{"RED":bool, "RED 2":bool, "RED 3":bool} {"RED"=FALSE, "RED 2"=FALSE, "RED 3"=TRUE} ("Ampel")) -> ()  [unwired: 2 in, 2 out]
                n286 = property on="YELLOW" class="Boolean (strict)"("Blinking"=FALSE) -> ()  [unwired: 2 in, 2 out]
              }
            }
          }
          event #6 {
            n287 = event-data() -> ()  [unwired: 1 in, 5 out]
          }
          event #7 {
            n288 = event-data() -> ()  [unwired: 1 in, 5 out]
            n289 = stacked-sequence {
              frame #0 {
              }
              frame #1 {
                n290 = control-ref of="Image Path"() -> (w317:refnum<vi>)
                n291 = call "GetSetTempDir.vi"("Path"=w317) -> ()  [unwired: 4 in]
              }
            }
          }
          event #8 {
            n292 = event-data() -> ()  [unwired: 1 in, 5 out]
            n293 = stacked-sequence {
              frame #0 {
                n294 = property on="Ampel" class="Clust (strict)"("Value"=cluster{"RED":bool, "RED 2":bool, "RED 3":bool} {"RED"=FALSE, "RED 2"=FALSE, "RED 3"=FALSE} ("Ampel")) -> ()  [unwired: 2 in, 2 out]
                n295 = property on="YELLOW" class="Boolean (strict)"("Blinking"=TRUE) -> ()  [unwired: 2 in, 2 out]
              }
              frame #1 {
                n296 = property on="Image LOADED" class="Bool (strict)"() -> ("Value"=w321:bool)  [unwired: 2 in, 2 out]
                n297 = case shown="True" w321 {
                  frame #0 {
                  }
                  frame #1 {
                    n298 = call "GetTACWindowIngoHeucke.vi"("Enum"=enum16{"ini", "get", "quick"}."ini") -> ("Cursor.Cursor Position:Cursor X"=w330:u16, "Cursor.Cursor Position:Cursor X 2"=w331:u16, "x-values"=w324:dbl[], "ready?"=w325:bool)  [unwired: 1 in, 5 out]
                    n299 = Select(t=2, s=w325, f=0) -> (s? t:f=w328:i32)
                    n300 = property on="TACwinLoaded?" class="Boolean (strict)"("Value"=TRUE ("TACwinLoaded?")) -> ()  [unwired: 2 in, 2 out]
                    n301 = call "CursorPositionChanged.vi"("CursorPos x1"=w331, "CursorPos x0"=w330, "x-values"=w324, "action"=enum16{"Check", "Get", "xval"}."xval" ("Enum")) -> ()  [unwired: 4 out]
                    n302 = property on="TAC Window" class="Boolean"("Disabled"=w328) -> ()  [unwired: 2 in, 2 out]
                  }
                }
              }
              frame #2 {
                n303 = property on="Ampel" class="Clust (strict)"("Value"=cluster{"RED":bool, "RED 2":bool, "RED 3":bool} {"RED"=FALSE, "RED 2"=FALSE, "RED 3"=TRUE} ("Ampel")) -> ()  [unwired: 2 in, 2 out]
                n304 = property on="YELLOW" class="Boolean (strict)"("Blinking"=FALSE) -> ()  [unwired: 2 in, 2 out]
                "Boolean" <- TRUE
              }
            }
          }
          event #9 {
            n305 = event-data() -> ()  [unwired: 1 in, 5 out]
          }
          event #10 {
            n306 = event-data() -> ()  [unwired: 1 in, 5 out]
            n307 = stacked-sequence {
              frame #0 {
              }
              frame #1 {
                n308 = control-ref of="Int duplex?"() -> (w341:refnum<vi>)
                n309 = control-ref of="16btimage?"() -> (w340:refnum<vi>)
                n310 = control-ref of="does a coinc image exist?"() -> (w339:refnum<vi>)
                n311 = control-ref of="Image Path"() -> (w338:refnum<vi>)
                n312 = control-ref of="notes"() -> (w337:refnum<vi>)
                n313 = call "ExportDialog.vi"("Int duplex ctl"=w341, "16 bit ctl"=w340, "coincidence image ctl"=w339, "Path"=w338, "notes 2"=w337) -> ()  [unwired: 4 in]
              }
            }
          }
          event #11 {
            n314 = event-data() -> ()  [unwired: 1 in, 5 out]
            n315 = stacked-sequence {
              frame #0 {
                n316 = property on="Ampel" class="Clust (strict)"("Value"=cluster{"RED":bool, "RED 2":bool, "RED 3":bool} {"RED"=FALSE, "RED 2"=FALSE, "RED 3"=FALSE} ("Ampel")) -> ()  [unwired: 2 in, 2 out]
                n317 = property on="YELLOW" class="Boolean (strict)"("Blinking"=TRUE) -> ()  [unwired: 2 in, 2 out]
              }
              frame #1 {
                n318 = property on="TACwinLoaded?" class="Bool (strict)"() -> ("Value"=w345:bool)  [unwired: 2 in, 2 out]
                n319 = case shown="False" w345 {
                  frame #0 {
                    n320 = call "GetTACWindowIngoHeucke.vi"("Enum"=enum16{"ini", "get", "quick"}."ini") -> ("Cursor.Cursor Position:Cursor X"=w349:u16, "Cursor.Cursor Position:Cursor X 2"=w348:u16, "x-values"=w347:dbl[])  [unwired: 1 in, 6 out]
                    n321 = call "CursorPositionChanged.vi"("CursorPos x1"=w348, "CursorPos x0"=w349, "x-values"=w347, "action"=enum16{"Check", "Get", "xval"}."xval" ("Enum")) -> ()  [unwired: 4 out]
                  }
                  frame #1 {
                  }
                }
              }
              frame #2 {
                n322 = property on="notes" class="String"() -> ("Value"=w352:string)  [unwired: 2 in, 2 out]
                n323 = Concatenate Strings(w352, "\n- F2 and lifetime image" ("string")) -> (w351:string)
                n324 = property on="notes" class="String"("Value"=w351) -> ()  [unwired: 2 in, 2 out]
              }
              frame #3 {
                n325 = property on="threshold" class="Clust (strict)"() -> ("Value"=w357:cluster{"max":u32, "min":u32})  [unwired: 2 in, 2 out]
                n326 = control-ref of="notes"() -> (w358:refnum<vi>)
                n327 = Unbundle(w357) -> ("max"=w356:u32, "min"=w355:u32)
                n328 = Max & Min(x=w356, y=w355) -> (min(x,y)=w354:u32)  [unwired: 1 out]
                n329 = control-ref of="Image Path"() -> (w359:refnum<vi>)
                n330 = call "ShowLifetimeAndF2Image.vi"("Path"=w359, "threshold (min)"=w354, "notes 2"=w358) -> ()  [unwired: 4 in]
              }
              frame #4 {
                n331 = property on="Ampel" class="Clust (strict)"("Value"=cluster{"RED":bool, "RED 2":bool, "RED 3":bool} {"RED"=FALSE, "RED 2"=FALSE, "RED 3"=TRUE} ("Ampel")) -> ()  [unwired: 2 in, 2 out]
                n332 = property on="YELLOW" class="Boolean (strict)"("Blinking"=FALSE) -> ()  [unwired: 2 in, 2 out]
              }
            }
          }
          event #12 {
            n333 = event-data() -> ()  [unwired: 1 in, 5 out]
            n334 = stacked-sequence {
              frame #0 {
                n335 = property on="16btimage?" class="Boolean (strict)"() -> ("Value"=w364:bool)  [unwired: 2 in, 2 out]
                n336 = Not(x=w364) -> (.not. x?=→"16btimage?":bool)
              }
              frame #1 {
                n337 = property on="16btimage?" class="Boolean (strict)"() -> ("Value"=w365:bool)  [unwired: 2 in, 2 out]
                n338 = case shown="True" w365 {
                  frame #0 {
                    n339 = call "16bitImageglobal.vi"("Enum"=T4."Dump") -> ()  [unwired: 4 in, 4 out]
                  }
                  frame #1 {
                    n340 = stacked-sequence {
                      frame #0 {
                        n341 = call "16bitImageglobal.vi"("Enum"=T4."Ini") -> ()  [unwired: 4 in, 4 out]
                      }
                      frame #1 {
                        n342 = property on="router" class="Ring (strict)"() -> ("Value"=w370:u8)  [unwired: 2 in, 2 out]
                        n343 = property on="plane" class="DigNum (strict)"() -> ("Value"=w369:u32)  [unwired: 2 in, 2 out]
                        n344 = call "16bitImageglobal.vi"("Enum"=T4."Input", "plane"=w369, "router"=w370) -> ()  [unwired: 2 in, 4 out]
                      }
                      frame #2 {
                        n345 = call "16bitImageglobal.vi"("Enum"=T4."Get") -> ()  [unwired: 4 in, 4 out]
                      }
                    }
                  }
                }
              }
            }
          }
          event #13 {
            n346 = event-data() -> ()  [unwired: 1 in, 5 out]
            n347 = stacked-sequence {
              frame #0 {
                n348 = property on="Ampel" class="Clust (strict)"("Value"=cluster{"RED":bool, "RED 2":bool, "RED 3":bool} {"RED"=FALSE, "RED 2"=FALSE, "RED 3"=FALSE} ("Ampel")) -> ()  [unwired: 2 in, 2 out]
                n349 = property on="YELLOW" class="Boolean (strict)"("Blinking"=TRUE) -> ()  [unwired: 2 in, 2 out]
                n350 = call "Intensityduplex.vi"("Enum"=T3."dump") -> ()  [unwired: 4 in, 2 out]
              }
              frame #1 {
                n351 = property on="notes" class="String"() -> ("Value"=w377:string)  [unwired: 2 in, 2 out]
                n352 = Concatenate Strings(w377, "\n- coincidence spotting" ("string")) -> (w376:string)
                n353 = property on="notes" class="String"("Value"=w376) -> ()  [unwired: 2 in, 2 out]
              }
              frame #2 {
                n354 = control-ref of="notes"() -> (w379:refnum<vi>)
                n355 = call "coincidenceImagenew.vi"("notes 2"=w379) -> ()  [unwired: 6 in]
              }
              frame #3 {
                n356 = property on="Ampel" class="Clust (strict)"("Value"=cluster{"RED":bool, "RED 2":bool, "RED 3":bool} {"RED"=FALSE, "RED 2"=FALSE, "RED 3"=TRUE} ("Ampel")) -> ()  [unwired: 2 in, 2 out]
                n357 = property on="YELLOW" class="Boolean (strict)"("Blinking"=FALSE) -> ()  [unwired: 2 in, 2 out]
              }
            }
          }
          event #14 {
            n358 = event-data() -> ()  [unwired: 1 in, 5 out]
            n359 = stacked-sequence {
              frame #0 {
                n360 = call "CoincidencePicture.vi"("Enum"=T6."Dump") -> ()  [unwired: 6 in, 3 out]
              }
              frame #1 {
                n361 = property on="notes" class="String"() -> ("Value"=w385:string)  [unwired: 2 in, 2 out]
                n362 = Concatenate Strings(w385, "\n- coincidence image" ("string")) -> (w384:string)
                n363 = property on="notes" class="String"("Value"=w384) -> ()  [unwired: 2 in, 2 out]
              }
              frame #2 {
                n364 = control-ref of="notes"() -> (w387:refnum<vi>)
                n365 = call "CoincidenceBuildImage.vi"("notes 2"=w387) -> ()  [unwired: 11 in]
              }
              frame #3 {
                n366 = call "CoincidencePicture.vi"("Enum"=enum16{"Ini", "Get", "Set", "Draw", "Colorpal"}."Get") -> ("String"=w390:string)  [unwired: 6 in, 2 out]
                n367 = Not Equal?(x=w390, y="") -> (x != y?=→"does a coinc image exist?":bool)
              }
            }
          }
          event #15 {
            n368 = event-data() -> ()  [unwired: 1 in, 5 out]
            n369 = stacked-sequence {
              frame #0 {
                n370 = call "ScanSubDirGlobal.vi"("set"=FALSE) -> ("Array"=w397:path[])  [unwired: 1 in]
                n371 = Index Array(array=w397, index="Header Path Ring") -> (element=w393:path)
                n372 = control-ref of="Image Path"() -> (w395:refnum<vi>)
                n373 = call "LoadHeaderKenandHerty.vi"("appended path"=w393, "reference"=w395) -> ("unsuccesful?"=w394:bool)  [unwired: 3 in]
                n374 = case shown="False" w394 {
                  tunnel: w393 -> [w399 _]
                  frame #0 {
                    n375 = call "FilePathGlobal.vi"("Image Path"=w399, "set?"=TRUE) -> ()  [unwired: 3 out]
                  }
                  frame #1 {
                  }
                }
              }
              frame #1 {
                n376 = control-ref of="notes"() -> (w401:refnum<vi>)
                n377 = control-ref of="Image Path"() -> (w403:refnum<vi>)
                n378 = call "SaveNotes.vi"("Enum"=enum16{"Get Path", "Read", "Save"}."Get Path", "String"=w401, "Path"=w403) -> ()  [unwired: 2 in]
              }
              frame #2 {
                w408 = u8 0 ("Disabled")
                n379 = property on="Load" class="Bool"("Visible"=FALSE) -> ()  [unwired: 2 in, 2 out]
                n380 = property on="Image LOADED" class="Boolean (strict)"("Disabled"=w408) -> ()  [unwired: 2 in, 2 out]
                n381 = property on="View Image Settings" class="Boolean"("Disabled"=w408) -> ()  [unwired: 2 in, 2 out]
                n382 = property on="View FIFO Settings" class="Boolean"("Disabled"=w408) -> ()  [unwired: 2 in, 2 out]
                n383 = property on="LOADED HDR" class="Bool (strict)"("Value"=TRUE ("Boolean")) -> ()  [unwired: 2 in, 2 out]
                n384 = property on="Ampel" class="Clust (strict)"("Value"=cluster{"RED":bool, "RED 2":bool, "RED 3":bool} {"RED"=TRUE, "RED 2"=TRUE, "RED 3"=FALSE} ("Ampel")) -> ()  [unwired: 2 in, 2 out]
                n385 = call "ViewImageSetnew.vi"("action"=enum16{"Display", "change", "Get", "Set"}."Get" ("Enum")) -> ("Image Settings"=w405:T10)  [unwired: 2 in]
                n386 = Unbundle By Name(w405) -> ("Retrace"=w406:bool)
                n387 = case shown="False" w406 {
                  frame #0 {
                    n388 = property on="Load Image" class="Boolean"("Disabled"=u8 0, "Visible"=TRUE) -> ()  [unwired: 2 in, 2 out]
                  }
                  frame #1 {
                    n389 = property on="Load Image" class="Boolean"("Disabled"=u8 2, "Visible"=FALSE) -> ()  [unwired: 2 in, 2 out]
                    n390 = One Button Dialog(message="Die Retrace kann derzeit noch nicht bearbeitet werden.") -> ()  [unwired: 1 in, 1 out]
                  }
                }
              }
              frame #3 {
                n391 = call "TempPath.vi"("change"=FALSE) -> ("stripped path 2"=w427:path)  [unwired: 2 in]
                n392 = Build Path(base path=w427, name or relative path="Anna_linescan.tmp" ("prompt")) -> (appended path=w425:path)
                n393 = property on="Image LOADED" class="Boolean (strict)"("Blinking"=TRUE) -> ()  [unwired: 2 in, 2 out]
                n394 = call <vilib>:"compatOverwrite.vi"("overwrite (F)"=TRUE) -> ("overwrite?"=w416:T13)
                n395 = Open/Create/Replace Datalog(5:T7 {"router"=[], "macro times"=[], "micro times"=[], "invalid"=[], "gap"=[]} ("cluster"), 10:w416, 11:w425) -> (3:w423:refnum<k1>)  [unwired: 3 in, 2 out]
                n396 = call "TempRefnum.vi"("change?"=TRUE, "refnum in"=w423) -> ()  [unwired: 1 out]
                n397 = property on="Header Path Ring" class="Ring (strict)"("Disabled"=u8 2) -> ()  [unwired: 2 in, 2 out]
                n398 = property on="Load Image" class="Boolean"("Disabled"=u8 2) -> ()  [unwired: 2 in, 2 out]
                n399 = call "sumofphotons.vi"("s"=TRUE, "sum of photons"=u32[][][][] []) -> ()  [unwired: 1 out]
              }
              frame #4 {
                n400 = control-ref of="Image Path"() -> (w430:refnum<vi>)
                n401 = call "fileformatGlobal.vi"("changed"=FALSE) -> ("fileformat out"=w432:enum16{"Herty", "Ken", "SPC130", "HydraHarp"})  [unwired: 1 in]
                n402 = case shown="\"Ken\"" w432 {
                  tunnel: w430 -> [w433 w434 w435]
                  frame #0 {
                    n403 = call "LoadData.vi"("Path"=w433) -> ()  [unwired: 2 in, 3 out]
                  }
                  frame #1 {
                    n404 = call "LoadDataSPC130.vi"("Path"=w434) -> ()  [unwired: 2 in, 3 out]
                  }
                  frame #2 {
                    n405 = call "LoadDataKen.vi"("Path"=w435) -> ()  [unwired: 5 in]
                  }
                }
              }
              frame #5 {
                n406 = stacked-sequence {
                  frame #0 {
                    n407 = call "TempRefnum.vi"("change?"=FALSE) -> ("refnum out"=w437:refnum<k1>)  [unwired: 1 in]
                    n408 = Close File(refnum=w437) -> (error out=w436:errorcluster)  [unwired: 1 in, 1 out]
                    n409 = call "HandleError.vi"("error in (no error)"=w436) -> ()
                  }
                  frame #1 {
                    n410 = call "TotalRecall_Reload.vi"() -> ("gap"=w439:i32, "invalid"=w440:i32, "valid"=w441:i32)  [unwired: 4 in, 1 out]
                    n411 = property on="total" class="DigNum (strict)"("Value"=w441) -> ()  [unwired: 2 in, 2 out]
                    n412 = property on="invalid" class="DigNum (strict)"("Value"=w440) -> ()  [unwired: 2 in, 2 out]
                    n413 = property on="gap" class="DigNum (strict)"("Value"=w439) -> ()  [unwired: 2 in, 2 out]
                  }
                  frame #2 {
                    n414 = call "sumofphotons.vi"("s"=FALSE) -> ("sum of photons out"=w443:u32[][][][])  [unwired: 1 in]
                    n415 = property on="plane" class="DigNum (strict)"() -> ("Value"=w446:u32)  [unwired: 2 in, 2 out]
                    n416 = property on="threshold" class="Clust (strict)"() -> ("Value"=w442:cluster{"max":u32, "min":u32})  [unwired: 2 in, 2 out]
                    n417 = property on="router" class="Ring (strict)"() -> ("Value"=w447:u8)  [unwired: 2 in, 2 out]
                    n418 = property on="RGB or false color?" class="Bool (strict)"() -> ("Value"=w448:bool)  [unwired: 2 in, 2 out]
                    n419 = call "OnlinePic.vi"("action"=T2."ini" ("Enum"), "RGB/False"=w448, "Threshold (max)"=w442, "plane"=w446, "router channel"=w447, "Array"=w443) -> ()  [unwired: 1 in, 5 out]
                  }
                  frame #3 {
                    n420 = call "ViewImageSetnew.vi"("action"=enum16{"Display", "change", "Get", "Set"}."Get" ("Enum")) -> ("Image Settings"=w452:T10)  [unwired: 2 in]
                    n421 = Unbundle By Name(w452) -> ("Image Size (pixel).z"=w451:u32)
                    n422 = case shown="0" w451 {
                      tunnel: [i8 2 w456] -> w450
                      tunnel: [u8 0 w456] -> w449
                      frame #0 {
                      }
                      frame #1 {
                        w456 = u8 0
                      }
                    }
                    n423 = property on="plane" class="DigNum (strict)"("Disabled"=w450, "Value"=w449) -> ()  [unwired: 2 in, 2 out]
                  }
                  frame #4 {
                    w457 = u8 0
                    n424 = property on="F2-Image" class="Boolean"("Disabled"=u8 0) -> ()  [unwired: 2 in, 2 out]
                    n425 = property on="Image LOADED" class="Boolean (strict)"("Blinking"=FALSE, "Value"=TRUE ("Image LOADED")) -> ()  [unwired: 2 in, 2 out]
                    n426 = property on="Lifetime pick" class="Boolean"("Disabled"=w457) -> ()  [unwired: 2 in, 2 out]
                    n427 = property on="RGB or false color?" class="Boolean (strict)"("Disabled"=w457) -> ()  [unwired: 2 in, 2 out]
                    n428 = property on="router" class="Ring (strict)"("Disabled"=w457) -> ()  [unwired: 2 in, 2 out]
                    n429 = property on="16bit" class="Boolean"("Disabled"=w457) -> ()  [unwired: 2 in, 2 out]
                    n430 = property on="threshold" class="Clust (strict)"("Disabled"=w457) -> ()  [unwired: 2 in, 2 out]
                    n431 = property on="coincidence spot" class="Boolean"("Disabled"=w457) -> ()  [unwired: 2 in, 2 out]
                    n432 = property on="TAC Window" class="Boolean"("Disabled"=w457) -> ()  [unwired: 2 in, 2 out]
                    n433 = property on="Export" class="Bool"("Disabled"=w457) -> ()  [unwired: 2 in, 2 out]
                    n434 = property on="coincidence\nimage" class="Bool"("Disabled"=w457) -> ()  [unwired: 2 in, 2 out]
                  }
                  frame #5 {
                    n435 = property on="Ampel" class="Clust (strict)"("Value"=cluster{"RED":bool, "RED 2":bool, "RED 3":bool} {"RED"=FALSE, "RED 2"=FALSE, "RED 3"=TRUE} ("Ampel")) -> ()  [unwired: 2 in, 2 out]
                  }
                }
              }
            }
          }
          event #16 {
            n436 = event-data() -> ("ItemTag"=w464:string)  [unwired: 1 in, 5 out]
            n437 = case shown="\"Spotfinder\"" w464 {
              tunnel: [_ _ TRUE _ _ _ _ _ _ _ _ _ _ _ _ _ _ _ _ _ _] -> w463
              frame #0 {
                n438 = control-ref of="Image Path"() -> (w465:refnum<vi>)
                n439 = property class="Path"(reference=w465) -> ("Value"=w466:path)  [unwired: 1 in, 2 out]
                n440 = Strip Path(path=w466) -> (stripped path=w467:path)  [unwired: 1 out]
                n441 = Not A Number/Path/Refnum?(number/path/refnum=w467) -> (NaN/Path/Refnum?=w468:bool)
                n442 = case shown="False" w468 {
                  tunnel: w467 -> [w471 _]
                  frame #0 {
                    n443 = call "fileformatGlobal.vi"() -> ("fileformat out"=w473:enum16{"Herty", "Ken", "SPC130", "HydraHarp"})  [unwired: 2 in]
                    n444 = case shown="\"SPC130\"" w473 {
                      tunnel: ["plane000line000.fifo" ("name or relative path") "plane000line000module000.spc" ("name or relative path") "0_0.ifif" ("name or relative path")] -> w472
                      frame #0 {
                      }
                      frame #1 {
                      }
                      frame #2 {
                      }
                    }
                    n445 = call "ViewFIFOSet.vi"("Enum"=enum16{"Display", "change", "Get", "Set"}."Get") -> ("FIFO Settings (Array)"=w479:T11[])  [unwired: 1 in]
                    n446 = Index Array(array=w479) -> (element=w469:T11)  [unwired: 1 in]
                    n447 = Unbundle By Name(w469) -> ("ADC.ADC Resolution"=w475:i32)
                    n448 = Not Equal To 0?(x=w475) -> (x != 0?=w474:bool)
                    n449 = Build Path(base path=w471, name or relative path=w472) -> (appended path=w470:path)
                    n450 = Select(t=enum16{"32 bit", "48 bit"}."48 bit" ("File Type"), s=w474, f=enum16{"32 bit", "48 bit"}."32 bit" ("File Type")) -> (s? t:f=w478:enum16{"32 bit", "48 bit"})
                    n451 = call "FIFORawDataScreener.vi"("File Type"=w478, "Path"=w470) -> ()  [unwired: 2 in]
                  }
                  frame #1 {
                    n452 = One Button Dialog(message="Select header file first!") -> ()  [unwired: 1 in, 1 out]
                  }
                }
              }
              frame #1 {
                n453 = call "ViewFIFOTrace.vi"() -> ()  [unwired: 1 in]
              }
              frame #2 {
              }
              frame #3 {
                n454 = stacked-sequence {
                  seq-local: [_ _ _ _ w519 _] -> [_ _ _ _ _ w531]
                  frame #0 {
                    n455 = control-ref of="notes"() -> (w490:refnum<vi>)
                    n456 = property class="Str"(reference=w490) -> (reference out=w486:refnum<vi>, "Value"=w488:string)  [unwired: 1 in, 1 out]
                    n457 = Not Equal?(x=w488, y="") -> (x != y?=w487:bool)
                    n458 = case shown="True" w487 {
                      tunnel: w486 -> [_ w491]
                      frame #0 {
                      }
                      frame #1 {
                        n459 = call "SaveNotes.vi"("Enum"=enum16{"Get Path", "Read", "Save"}."Save", "String"=w491) -> ()  [unwired: 3 in]
                      }
                    }
                  }
                  frame #1 {
                    w507 = FALSE ("Boolean")
                    w500 = u8 2 ("Disabled")
                    n460 = property on="TACwinLoaded?" class="Boolean (strict)"("Value"=FALSE ("TACwinLoaded?")) -> ()  [unwired: 2 in, 2 out]
                    n461 = property on="F2-Image" class="Boolean"("Disabled"=u8 2) -> ()  [unwired: 2 in, 2 out]
                    n462 = property on="TAC Window" class="Boolean"("Disabled"=2) -> ()  [unwired: 2 in, 2 out]
                    n463 = property on="LOADED HDR" class="Bool (strict)"("Value"=w507) -> ()  [unwired: 2 in, 2 out]
                    n464 = property on="Image LOADED" class="Boolean (strict)"("Value"=w507, "Blinking"=FALSE) -> ()  [unwired: 2 in, 2 out]
                    n465 = property on="Image Path" class="Path"("Disabled"=u8 0) -> ()  [unwired: 2 in, 2 out]
                    n466 = property on="Load" class="Bool"("Visible"=TRUE) -> ()  [unwired: 2 in, 2 out]
                    n467 = property on="RGB or false color?" class="Boolean (strict)"("Disabled"=w500, "Value"=w507) -> ()  [unwired: 2 in, 2 out]
                    n468 = property on="Lifetime pick" class="Boolean"("Disabled"=w500) -> ()  [unwired: 2 in, 2 out]
                    n469 = property on="router" class="Ring (strict)"("Disabled"=w500) -> ()  [unwired: 2 in, 2 out]
                    n470 = property on="plane" class="DigNum (strict)"("Disabled"=w500) -> ()  [unwired: 2 in, 2 out]
                    n471 = property on="Export" class="Boolean"("Disabled"=w500) -> ()  [unwired: 2 in, 2 out]
                    n472 = property on="View Image Settings" class="Boolean"("Disabled"=w500) -> ()  [unwired: 2 in, 2 out]
                    n473 = property on="View FIFO Settings" class="Boolean"("Disabled"=w500) -> ()  [unwired: 2 in, 2 out]
                    n474 = property on="Load Image" class="Boolean"("Disabled"=w500, "Visible"=FALSE) -> ()  [unwired: 2 in, 2 out]
                    n475 = property on="16bit" class="Boolean"("Disabled"=w500) -> ()  [unwired: 2 in, 2 out]
                    n476 = property on="Spotfinder" class="Boolean"("Disabled"=w500) -> ()  [unwired: 2 in, 2 out]
                    n477 = property on="notes" class="String"("Value"="") -> ()  [unwired: 2 in, 2 out]
                    n478 = property on="invalid" class="DigNum (strict)"("Value"=u32 0 ("invalid photons")) -> ()  [unwired: 2 in, 2 out]
                    n479 = property on="gap" class="DigNum (strict)"("Value"=u32 0 ("gap photons")) -> ()  [unwired: 2 in, 2 out]
                    n480 = property on="total" class="DigNum (strict)"("Value"=u32 0 ("invalid photons")) -> ()  [unwired: 2 in, 2 out]
                    n481 = call "sumofphotons.vi"("s"=TRUE, "sum of photons"=u32[][][][] []) -> ()  [unwired: 1 out]
                  }
                  frame #2 {
                    n482 = call "IMAQ WindClose"("Close All Windows (False)"=TRUE ("Close All Windows (N)")) -> ("error out"=w514:errorcluster)  [unwired: 5 in]
                    n483 = call "IMAQ Dispose"("All Images? (No)"=TRUE, "error in (no error)"=w514) -> ("error out"=w515:errorcluster)  [unwired: 4 in]
                    n484 = call "IMAQ WindToolsClose"("error in (no error)"=w515) -> ("error out"=w508:errorcluster)  [unwired: 5 in]
                    n485 = call "Intensityduplex.vi"("Enum"=T3."dump") -> ()  [unwired: 4 in, 2 out]
                    n486 = call "OnlinePic.vi"("action"=T2."clear" ("Enum")) -> ()  [unwired: 6 in, 5 out]
                    n487 = call "16bitImageglobal.vi"("Enum"=T4."Ini") -> ()  [unwired: 4 in, 4 out]
                    n488 = call "HandleError.vi"("error in (no error)"=w508) -> ()
                    n489 = Wait Until Next ms Multiple(millisecond multiple=u32 2500) -> ()  [unwired: 1 out]
                  }
                  frame #3 {
                    n490 = property on="Ampel" class="Clust (strict)"("Value"=cluster{"RED":bool, "RED 2":bool, "RED 3":bool} {"RED"=TRUE, "RED 2"=FALSE, "RED 3"=FALSE} ("Ampel")) -> ()  [unwired: 2 in, 2 out]
                  }
                  frame #4 {
                    (unwired) T9."existing file" ("select mode (2)")
                    n491 = File Dialog(6:"*.hdr; fileinfo.txt" ("pattern"), 7:"Select header file ... (quick view)" ("prompt")) -> (0:w518:errorcluster, 1:w520:bool, 3:w521:path)  [unwired: 5 in, 1 out]
                    n492 = Unbundle(w518) -> ()  [unwired: 3 out]
                    n493 = case shown="False" w520 {
                      tunnel: w521 -> [w526 _]
                      tunnel: [1 0] -> w519
                      frame #0 {
                        n494 = control-ref of="Image Path"() -> (w525:refnum<vi>)
                        n495 = call "LoadHeaderKenandHerty.vi"("appended path"=w526, "reference"=w525) -> ()  [unwired: 3 in, 1 out]
                        n496 = Path To String(path=w526) -> (string=w527:string)
                        n497 = Concatenate Strings("Anna_linescan " ("string"), w527) -> (w529:string)
                        n498 = property class="VI"("Front Panel Window:Title"=w529) -> ()  [unwired: 2 in, 2 out]
                      }
                      frame #1 {
                      }
                    }
                  }
                  frame #5 {
                    n499 = for {
                      N: w531 -> [_]
                      n500 = stacked-sequence {
                        frame #0 {
                          w532 = u8 0 ("Disabled")
                          n501 = property on="LOADED HDR" class="Bool (strict)"("Value"=TRUE ("Boolean")) -> ()  [unwired: 2 in, 2 out]
                          n502 = property on="Load" class="Bool"("Visible"=FALSE) -> ()  [unwired: 2 in, 2 out]
                          n503 = property on="Image LOADED" class="Boolean (strict)"("Disabled"=w532) -> ()  [unwired: 2 in, 2 out]
                          n504 = property on="View Image Settings" class="Boolean"("Disabled"=w532) -> ()  [unwired: 2 in, 2 out]
                          n505 = property on="View FIFO Settings" class="Boolean"("Disabled"=w532) -> ()  [unwired: 2 in, 2 out]
                          n506 = control-ref of="notes"() -> (w538:refnum<vi>)
                          n507 = control-ref of="Image Path"() -> (w536:refnum<vi>)
                          n508 = property on="Ampel" class="Clust (strict)"("Value"=cluster{"RED":bool, "RED 2":bool, "RED 3":bool} {"RED"=TRUE, "RED 2"=TRUE, "RED 3"=FALSE} ("Ampel")) -> ()  [unwired: 2 in, 2 out]
                          n509 = call "SaveNotes.vi"("Enum"=enum16{"Get Path", "Read", "Save"}."Get Path", "String"=w538, "Path"=w536) -> ()  [unwired: 2 in]
                        }
                        frame #1 {
                          n510 = call "ViewImageSetnew.vi"("action"=enum16{"Display", "change", "Get", "Set"}."Get" ("Enum")) -> ("Image Settings"=w540:T10)  [unwired: 2 in]
                          n511 = Unbundle By Name(w540) -> ("Retrace"=w539:bool)
                          n512 = case shown="False" w539 {
                            frame #0 {
                              n513 = property on="Load Image" class="Boolean"("Disabled"=u8 0, "Visible"=TRUE) -> ()  [unwired: 2 in, 2 out]
                            }
                            frame #1 {
                              n514 = property on="Load Image" class="Boolean"("Disabled"=u8 2, "Visible"=FALSE) -> ()  [unwired: 2 in, 2 out]
                              n515 = One Button Dialog(message="Die Retrace kann derzeit noch nicht bearbeitet werden.") -> ()  [unwired: 1 in, 1 out]
                            }
                          }
                        }
                        frame #2 {
                          n516 = property on="Image Path" class="Path"("Disabled"=u8 2) -> ()  [unwired: 2 in, 2 out]
                          n517 = property on="Load Image" class="Boolean"("Disabled"=u8 2) -> ()  [unwired: 2 in, 2 out]
                          n518 = property on="Image LOADED" class="Boolean (strict)"("Blinking"=TRUE) -> ()  [unwired: 2 in, 2 out]
                          n519 = call "sumofphotons.vi"("s"=TRUE, "sum of photons"=u32[][][][] []) -> ()  [unwired: 1 out]
                        }
                        frame #3 {
                          n520 = control-ref of="Image Path"() -> (w556:refnum<vi>)
                          n521 = call "fileformatGlobal.vi"() -> ("fileformat out"=w555:enum16{"Herty", "Ken", "SPC130", "HydraHarp"})  [unwired: 2 in]
                          n522 = call "QuickLoadData.vi"("Fileformat"=w555, "Path"=w556) -> ("gap photons"=w552:u32, "invalid photons"=w554:u32, "total"=w553:u32)  [unwired: 1 in]
                          n523 = property on="invalid" class="DigNum (strict)"("Value"=w553) -> ()  [unwired: 2 in, 2 out]
                          n524 = property on="total" class="DigNum (strict)"("Value"=w554) -> ()  [unwired: 2 in, 2 out]
                          n525 = property on="gap" class="DigNum (strict)"("Value"=w552) -> ()  [unwired: 2 in, 2 out]
                        }
                        frame #4 {
                          n526 = call "sumofphotons.vi"("s"=FALSE) -> ("sum of photons out"=w559:u32[][][][])  [unwired: 1 in]
                          n527 = property on="threshold" class="Clust (strict)"() -> ("Value"=w557:cluster{"max":u32, "min":u32})  [unwired: 2 in, 2 out]
                          n528 = property on="router" class="Ring (strict)"() -> ("Value"=w562:u8)  [unwired: 2 in, 2 out]
                          n529 = property on="plane" class="DigNum (strict)"() -> ("Value"=w563:u32)  [unwired: 2 in, 2 out]
                          n530 = property on="RGB or false color?" class="Bool (strict)"() -> ("Value"=w561:bool)  [unwired: 2 in, 2 out]
                          n531 = call "OnlinePic.vi"("action"=T2."ini" ("Enum"), "RGB/False"=w561, "Threshold (max)"=w557, "plane"=w563, "router channel"=w562, "Array"=w559) -> ()  [unwired: 1 in, 5 out]
                        }
                        frame #5 {
                          n532 = call "ViewImageSetnew.vi"("action"=enum16{"Display", "change", "Get", "Set"}."Get" ("Enum")) -> ("Image Settings"=w565:T10)  [unwired: 2 in]
                          n533 = Unbundle By Name(w565) -> ("Image Size (pixel).z"=w566:u32)
                          n534 = case shown="0" w566 {
                            tunnel: [i8 2 w571] -> w567
                            tunnel: [u8 0 w571] -> w568
                            frame #0 {
                            }
                            frame #1 {
                              w571 = u8 0
                            }
                          }
                          n535 = property on="plane" class="DigNum (strict)"("Disabled"=w567, "Value"=w568) -> ()  [unwired: 2 in, 2 out]
                        }
                        frame #6 {
                          w572 = u8 0
                          w573 = u8 2 ("Disabled")
                          n536 = property on="Image LOADED" class="Boolean (strict)"("Blinking"=FALSE, "Value"=TRUE ("Image LOADED")) -> ()  [unwired: 2 in, 2 out]
                          n537 = property on="Lifetime pick" class="Boolean"("Disabled"=w573) -> ()  [unwired: 2 in, 2 out]
                          n538 = property on="TAC Window" class="Boolean"("Disabled"=w573) -> ()  [unwired: 2 in, 2 out]
                          n539 = property on="coincidence spot" class="Boolean"("Disabled"=w573) -> ()  [unwired: 2 in, 2 out]
                          n540 = property on="coincidence\nimage" class="Bool"("Disabled"=w573) -> ()  [unwired: 2 in, 2 out]
                          n541 = property on="RGB or false color?" class="Boolean (strict)"("Disabled"=w572) -> ()  [unwired: 2 in, 2 out]
                          n542 = property on="router" class="Ring (strict)"("Disabled"=w572) -> ()  [unwired: 2 in, 2 out]
                          n543 = property on="16bit" class="Boolean"("Disabled"=w572) -> ()  [unwired: 2 in, 2 out]
                          n544 = property on="Export" class="Bool"("Disabled"=w572) -> ()  [unwired: 2 in, 2 out]
                          n545 = property on="threshold" class="Clust (strict)"("Disabled"=w572) -> ()  [unwired: 2 in, 2 out]
                        }
                        frame #7 {
                          n546 = property on="Ampel" class="Clust (strict)"("Value"=cluster{"RED":bool, "RED 2":bool, "RED 3":bool} {"RED"=FALSE, "RED 2"=FALSE, "RED 3"=TRUE} ("Ampel")) -> ()  [unwired: 2 in, 2 out]
                        }
                      }
                    }
                  }
                }
              }
              frame #4 {
                n547 = stacked-sequence {
                  seq-local: [_ w590 _] -> [_ _ w602]
                  frame #0 {
                    n548 = property on="LOADED HDR" class="Boolean (strict)"() -> ("Value"=w584:bool)  [unwired: 2 in, 2 out]
                    n549 = case shown="True" w584 {
                      frame #0 {
                      }
                      frame #1 {
                        w588 = FALSE ("Boolean")
                        w587 = u8 2 ("Disabled")
                        n550 = property on="Image LOADED" class="Boolean (strict)"("Value"=w588, "Blinking"=w588) -> ()  [unwired: 2 in, 2 out]
                        n551 = property on="Spotfinder" class="Boolean"("Disabled"=w587) -> ()  [unwired: 2 in, 2 out]
                        n552 = property on="TAC Window" class="Boolean"("Disabled"=w587) -> ()  [unwired: 2 in, 2 out]
                        n553 = property on="Export" class="Boolean"("Disabled"=w587) -> ()  [unwired: 2 in, 2 out]
                        n554 = property on="View Image Settings" class="Boolean"("Disabled"=w587) -> ()  [unwired: 2 in, 2 out]
                        n555 = property on="View FIFO Settings" class="Boolean"("Disabled"=w587) -> ()  [unwired: 2 in, 2 out]
                      }
                    }
                    n556 = control-ref of="notes"() -> (w577:refnum<vi>)
                    n557 = property class="Str"(reference=w577) -> (reference out=w578:refnum<vi>, "Value"=w580:string)  [unwired: 1 in, 1 out]
                    n558 = Not Equal?(x=w580, y="") -> (x != y?=w579:bool)
                    n559 = case shown="True" w579 {
                      tunnel: w578 -> [_ w585]
                      frame #0 {
                      }
                      frame #1 {
                        n560 = call "SaveNotes.vi"("Enum"=enum16{"Get Path", "Read", "Save"}."Save", "String"=w585) -> ()  [unwired: 3 in]
                      }
                    }
                    n561 = call "Intensityduplex.vi"("Enum"=T3."dump") -> ()  [unwired: 4 in, 2 out]
                    n562 = call "OnlinePic.vi"("action"=T2."clear" ("Enum")) -> ()  [unwired: 6 in, 5 out]
                  }
                  frame #1 {
                    (unwired) T9."existing file" ("select mode (2)")
                    n563 = File Dialog(6:"*.hdr; fileinfo.txt" ("pattern"), 7:"Select header file ..." ("prompt")) -> (0:w589:errorcluster, 1:w594:bool, 3:w593:path)  [unwired: 5 in, 1 out]
                    n564 = Unbundle(w589) -> ()  [unwired: 3 out]
                    n565 = case shown="False" w594 {
                      tunnel: w593 -> [w596 _]
                      tunnel: [1 0] -> w590
                      frame #0 {
                        n566 = control-ref of="Image Path"() -> (w597:refnum<vi>)
                        n567 = Path To String(path=w596) -> (string=w598:string)
                        n568 = call "LoadHeaderKenandHerty.vi"("appended path"=w596, "reference"=w597) -> ()  [unwired: 3 in, 1 out]
                        n569 = Concatenate Strings("Anna_linescan " ("string"), w598) -> (w600:string)
                        n570 = property class="VI"("Front Panel Window:Title"=w600) -> ()  [unwired: 2 in, 2 out]
                      }
                      frame #1 {
                      }
                    }
                  }
                  frame #2 {
                    n571 = for {
                      N: w602 -> [_]
                      n572 = stacked-sequence {
                        frame #0 {
                          w610 = u8 0 ("Disabled")
                          n573 = property on="Image LOADED" class="Boolean (strict)"("Disabled"=w610) -> ()  [unwired: 2 in, 2 out]
                          n574 = property on="View Image Settings" class="Boolean"("Disabled"=w610) -> ()  [unwired: 2 in, 2 out]
                          n575 = property on="View FIFO Settings" class="Boolean"("Disabled"=w610) -> ()  [unwired: 2 in, 2 out]
                          n576 = property on="LOADED HDR" class="Bool (strict)"("Value"=TRUE ("Boolean")) -> ()  [unwired: 2 in, 2 out]
                          n577 = control-ref of="notes"() -> (w603:refnum<vi>)
                          n578 = control-ref of="Image Path"() -> (w605:refnum<vi>)
                          n579 = property on="Ampel" class="Clust (strict)"("Value"=cluster{"RED":bool, "RED 2":bool, "RED 3":bool} {"RED"=TRUE, "RED 2"=TRUE, "RED 3"=FALSE} ("Ampel")) -> ()  [unwired: 2 in, 2 out]
                          n580 = call "SaveNotes.vi"("Enum"=enum16{"Get Path", "Read", "Save"}."Get Path", "String"=w603, "Path"=w605) -> ()  [unwired: 2 in]
                          n581 = call "ViewImageSetnew.vi"("action"=enum16{"Display", "change", "Get", "Set"}."Get" ("Enum")) -> ("Image Settings"=w607:T10)  [unwired: 2 in]
                          n582 = Unbundle By Name(w607) -> ("Retrace"=w608:bool)
                          n583 = property on="Load" class="Bool"("Visible"=FALSE) -> ()  [unwired: 2 in, 2 out]
                          n584 = case shown="False" w608 {
                            frame #0 {
                              n585 = property on="Load Image" class="Boolean"("Disabled"=u8 0, "Visible"=TRUE) -> ()  [unwired: 2 in, 2 out]
                            }
                            frame #1 {
                              n586 = property on="Load Image" class="Boolean"("Disabled"=u8 2, "Visible"=FALSE) -> ()  [unwired: 2 in, 2 out]
                              n587 = One Button Dialog(message="Die Retrace kann derzeit noch nicht bearbeitet werden.") -> ()  [unwired: 1 in, 1 out]
                            }
                          }
                        }
                        frame #1 {
                          n588 = property on="Image LOADED" class="Boolean (strict)"("Blinking"=TRUE) -> ()  [unwired: 2 in, 2 out]
                          n589 = property on="Image Path" class="Path"("Disabled"=u8 2) -> ()  [unwired: 2 in, 2 out]
                          n590 = property on="Load Image" class="Boolean"("Disabled"=u8 2) -> ()  [unwired: 2 in, 2 out]
                          n591 = call "sumofphotons.vi"("s"=TRUE, "sum of photons"=u32[][][][] []) -> ()  [unwired: 1 out]
                        }
                        frame #2 {
                          n592 = call "TempPath.vi"("change"=FALSE) -> ("stripped path 2"=w626:path)  [unwired: 2 in]
                          n593 = Build Path(base path=w626, name or relative path="Anna_linescan.tmp" ("prompt")) -> (appended path=w628:path)
                          n594 = call <vilib>:"compatOverwrite.vi"("overwrite (F)"=TRUE) -> ("overwrite?"=w623:T13)
                          n595 = Open/Create/Replace Datalog(5:T7 {"router"=[], "macro times"=[], "micro times"=[], "invalid"=[], "gap"=[]} ("cluster"), 10:w623, 11:w628) -> (3:w631:refnum<k1>)  [unwired: 3 in, 2 out]
                          n596 = call "TempRefnum.vi"("change?"=TRUE, "refnum in"=w631) -> ()  [unwired: 1 out]
                        }
                        frame #3 {
                          n597 = property on="LOADED HDR" class="Bool (strict)"() -> ("Value"=w632:bool)  [unwired: 2 in, 2 out]
                          n598 = case shown="True" w632 {
                            frame #0 {
                            }
                            frame #1 {
                              n599 = control-ref of="Image Path"() -> (w634:refnum<vi>)
                              n600 = call "fileformatGlobal.vi"() -> ("fileformat out"=w633:enum16{"Herty", "Ken", "SPC130", "HydraHarp"})  [unwired: 2 in]
                              n601 = case shown="\"Ken\"" w633 {
                                tunnel: w634 -> [w635 w636 w637]
                                frame #0 {
                                n602 = call "LoadDataSPC130.vi"("Path"=w635) -> ()  [unwired: 2 in, 3 out]
                                }
                                frame #1 {
                                n603 = call "LoadData.vi"("Path"=w636) -> ()  [unwired: 2 in, 3 out]
                                }
                                frame #2 {
                                n604 = call "LoadDataKen.vi"("Path"=w637) -> ()  [unwired: 5 in]
                                }
                              }
                            }
                          }
                        }
                        frame #4 {
                          n605 = call "TempRefnum.vi"("change?"=FALSE) -> ("refnum out"=w639:refnum<k1>)  [unwired: 1 in]
                          n606 = Close File(refnum=w639) -> (error out=w638:errorcluster)  [unwired: 1 in, 1 out]
                          n607 = call "HandleError.vi"("error in (no error)"=w638) -> ()
                        }
                        frame #5 {
                          n608 = call "TotalRecall_Reload.vi"() -> ("gap"=w641:i32, "invalid"=w642:i32, "valid"=w643:i32)  [unwired: 4 in, 1 out]
                          n609 = property on="total" class="DigNum (strict)"("Value"=w643) -> ()  [unwired: 2 in, 2 out]
                          n610 = property on="invalid" class="DigNum (strict)"("Value"=w642) -> ()  [unwired: 2 in, 2 out]
                          n611 = property on="gap" class="DigNum (strict)"("Value"=w641) -> ()  [unwired: 2 in, 2 out]
                        }
                        frame #6 {
                          n612 = call "sumofphotons.vi"("s"=FALSE) -> ("sum of photons out"=w645:u32[][][][])  [unwired: 1 in]
                          n613 = property on="router" class="Ring (strict)"() -> ("Value"=w649:u8)  [unwired: 2 in, 2 out]
                          n614 = property on="plane" class="DigNum (strict)"() -> ("Value"=w648:u32)  [unwired: 2 in, 2 out]
                          n615 = property on="threshold" class="Clust (strict)"() -> ("Value"=w644:cluster{"max":u32, "min":u32})  [unwired: 2 in, 2 out]
                          n616 = property on="RGB or false color?" class="Bool (strict)"() -> ("Value"=w650:bool)  [unwired: 2 in, 2 out]
                          n617 = call "OnlinePic.vi"("action"=T2."ini" ("Enum"), "RGB/False"=w650, "Threshold (max)"=w644, "plane"=w648, "router channel"=w649, "Array"=w645) -> ()  [unwired: 1 in, 5 out]
                        }
                        frame #7 {
                          n618 = call "ViewImageSetnew.vi"("action"=enum16{"Display", "change", "Get", "Set"}."Get" ("Enum")) -> ("Image Settings"=w652:T10)  [unwired: 2 in]
                          n619 = Unbundle By Name(w652) -> ("Image Size (pixel).z"=w653:u32)
                          n620 = case shown="0" w653 {
                            tunnel: [i8 2 w658] -> w654
                            tunnel: [u8 0 w658] -> w655
                            frame #0 {
                            }
                            frame #1 {
                              w658 = u8 0
                            }
                          }
                          n621 = property on="plane" class="DigNum (strict)"("Disabled"=w654, "Value"=w655) -> ()  [unwired: 2 in, 2 out]
                        }
                        frame #8 {
                          w660 = u8 0 ("Disabled")
                          w659 = u8 0
                          n622 = property on="Image LOADED" class="Boolean (strict)"("Blinking"=FALSE, "Value"=TRUE ("Image LOADED")) -> ()  [unwired: 2 in, 2 out]
                          n623 = property on="Lifetime pick" class="Boolean"("Disabled"=w659) -> ()  [unwired: 2 in, 2 out]
                          n624 = property on="RGB or false color?" class="Boolean (strict)"("Disabled"=w659) -> ()  [unwired: 2 in, 2 out]
                          n625 = property on="router" class="Ring (strict)"("Disabled"=w659) -> ()  [unwired: 2 in, 2 out]
                          n626 = property on="16bit" class="Boolean"("Disabled"=w659) -> ()  [unwired: 2 in, 2 out]
                          n627 = property on="threshold" class="Clust (strict)"("Disabled"=w659) -> ()  [unwired: 2 in, 2 out]
                          n628 = property on="coincidence spot" class="Boolean"("Disabled"=w659) -> ()  [unwired: 2 in, 2 out]
                          n629 = property on="F2-Image" class="Boolean"("Disabled"=w660) -> ()  [unwired: 2 in, 2 out]
                          n630 = property on="TAC Window" class="Boolean"("Disabled"=w659) -> ()  [unwired: 2 in, 2 out]
                          n631 = property on="Export" class="Bool"("Disabled"=w659) -> ()  [unwired: 2 in, 2 out]
                          n632 = property on="Spotfinder" class="Boolean"("Disabled"=w660) -> ()  [unwired: 2 in, 2 out]
                          n633 = property on="coincidence\nimage" class="Bool"("Disabled"=w659) -> ()  [unwired: 2 in, 2 out]
                        }
                        frame #9 {
                          n634 = property on="Ampel" class="Clust (strict)"("Value"=cluster{"RED":bool, "RED 2":bool, "RED 3":bool} {"RED"=FALSE, "RED 2"=FALSE, "RED 3"=TRUE} ("Ampel")) -> ()  [unwired: 2 in, 2 out]
                        }
                      }
                    }
                  }
                }
              }
              frame #5 {
                n635 = property on="Image Path" class="Path"() -> ("Value"=w664:path)  [unwired: 2 in, 2 out]
                n636 = call "imagemanipulation.vi"("Results"=w664) -> ()  [unwired: 7 in]
              }
              frame #6 {
                n637 = stacked-sequence {
                  frame #0 {
                    n638 = property on="Ampel" class="Clust (strict)"("Value"=cluster{"RED":bool, "YELLOW":bool, "GREEN":bool} {"RED"=FALSE, "YELLOW"=FALSE, "GREEN"=FALSE} ("Ampel")) -> ("Controls[]"=w666:refnum<vi>[])  [unwired: 2 in, 2 out]
                    n639 = Index Array(array=w666, index=1) -> (element=w668:refnum<vi>)
                    n640 = property class="Ctl"(reference=w668, "Blinking"=TRUE) -> ()  [unwired: 1 in, 2 out]
                  }
                  frame #1 {
                    n641 = control-ref of="notes"() -> ()  [unwired: 1 out]
                  }
                  frame #2 {
                    n642 = property on="Ampel" class="Clust (strict)"("Value"=cluster{"RED":bool, "YELLOW":bool, "GREEN":bool} {"RED"=FALSE, "YELLOW"=FALSE, "GREEN"=TRUE} ("Ampel")) -> ("Controls[]"=w673:refnum<vi>[])  [unwired: 2 in, 2 out]
                    n643 = Index Array(array=w673, index=1) -> (element=w671:refnum<vi>)
                    n644 = property class="Ctl"(reference=w671, "Blinking"=FALSE) -> ()  [unwired: 1 in, 2 out]
                  }
                }
              }
              frame #7 {
                n645 = control-ref of="Image Path"() -> (w675:refnum<vi>)
                n646 = control-ref of="notes"() -> (w676:refnum<vi>)
                n647 = call "TimeGatedImage.vi"("Image Path"=w675, "notes 3"=w676) -> ()  [unwired: 2 in]
              }
              frame #8 {
                n648 = call "Splashscreen.vi"("Mode"=enum16{"splash", "dialog"}."dialog") -> ()  [unwired: 1 in]
              }
              frame #9 {
                n649 = call "ViewFIFOSet.vi"("Enum"=enum16{"Display", "change", "Get", "Set"}."Display") -> ()  [unwired: 1 in, 1 out]
              }
              frame #10 {
                n650 = call "ViewImageSetnew.vi"("action"=enum16{"Display", "change", "Get", "Set"}."Display" ("Enum")) -> ()  [unwired: 2 in, 1 out]
              }
              frame #11 {
                n651 = control-ref of="Image Path"() -> (w680:refnum<vi>)
                n652 = call "GetSetTempDir.vi"("Path"=w680) -> ()  [unwired: 4 in]
              }
              frame #12 {
                n653 = control-ref of="Int duplex?"() -> (w685:refnum<vi>)
                n654 = control-ref of="16btimage?"() -> (w684:refnum<vi>)
                n655 = control-ref of="does a coinc image exist?"() -> (w683:refnum<vi>)
                n656 = control-ref of="Image Path"() -> (w681:refnum<vi>)
                n657 = control-ref of="notes"() -> (w682:refnum<vi>)
                n658 = call "ExportDialog.vi"("Int duplex ctl"=w685, "16 bit ctl"=w684, "coincidence image ctl"=w683, "Path"=w681, "notes 2"=w682) -> ()  [unwired: 4 in]
              }
              frame #13 {
                n659 = while {
                  stop <- w686 stop-if-true
                  n660 = property on="Image LOADED" class="Bool (strict)"() -> ("Value"=w686:bool)  [unwired: 2 in, 2 out]
                  n661 = case shown="True" w686 {
                    frame #0 {
                      n662 = while {
                        shift-right: [w689] -> _
                        shift-left: 9 -> [w690]
                        stop <- w688 stop-if-true
                        n663 = case shown="4" w690 {
                          tunnel: [1 2 3 4 10 6 7 8 _ _ _] -> w689
                          tunnel: [w696 _ _ _ _ _ _ _ _ _ _] -> w688
                          frame #0 {
                            n664 = while {
                              tunnel: [w703] -> w691
                              tunnel: [w699] -> w696
                              stop <- w700 continue-if-true
                              (unwired) T9."existing file" ("select mode (2)")
                              n665 = File Dialog(6:"*.hdr; fileinfo.txt" ("pattern"), 7:"Select header file" ("prompt")) -> (0:w698:errorcluster, 1:w699:bool, 3:w703:path)  [unwired: 5 in, 1 out]
                              n666 = Unbundle(w698) -> ()  [unwired: 3 out]
                              n667 = Not(x=w699) -> (.not. x?=w702:bool)
                              n668 = Not A Number/Path/Refnum?(number/path/refnum=w703) -> (NaN/Path/Refnum?=w701:bool)
                              n669 = And(x=w702, y=w701) -> (x .and. y?=w700:bool)
                            }
                            n670 = control-ref of="Image Path"() -> (w695:refnum<vi>)
                            n671 = Path To String(path=w691) -> (string=w694:string)
                            n672 = call "LoadHeaderKenandHerty.vi"("appended path"=w691, "reference"=w695) -> ()  [unwired: 3 in, 1 out]
                            n673 = Concatenate Strings("Anna_linescan " ("string"), w694) -> (w692:string)
                            n674 = property class="VI"("Front Panel Window:Title"=w692) -> ()  [unwired: 2 in, 2 out]
                          }
                          frame #1 {
                            w707 = u8 0 ("Disabled")
                            n675 = property on="Load" class="Bool"("Visible"=FALSE) -> ()  [unwired: 2 in, 2 out]
                            n676 = property on="LOADED HDR" class="Bool (strict)"("Value"=TRUE ("Boolean")) -> ()  [unwired: 2 in, 2 out]
                            n677 = property on="Image LOADED" class="Boolean (strict)"("Disabled"=w707) -> ()  [unwired: 2 in, 2 out]
                            n678 = property on="View Image Settings" class="Boolean"("Disabled"=w707) -> ()  [unwired: 2 in, 2 out]
                            n679 = property on="View FIFO Settings" class="Boolean"("Disabled"=w707) -> ()  [unwired: 2 in, 2 out]
                            n680 = property on="Ampel" class="Clust (strict)"("Value"=cluster{"RED":bool, "RED 2":bool, "RED 3":bool} {"RED"=TRUE, "RED 2"=TRUE, "RED 3"=FALSE} ("Ampel")) -> ()  [unwired: 2 in, 2 out]
                            n681 = call "ViewImageSetnew.vi"("action"=enum16{"Display", "change", "Get", "Set"}."Get" ("Enum")) -> ("Image Settings"=w715:T10)  [unwired: 2 in]
                            n682 = control-ref of="notes"() -> (w713:refnum<vi>)
                            n683 = control-ref of="Image Path"() -> (w711:refnum<vi>)
                            n684 = Unbundle By Name(w715) -> ("Retrace"=w714:bool)
                            n685 = call "SaveNotes.vi"("Enum"=enum16{"Get Path", "Read", "Save"}."Get Path", "String"=w713, "Path"=w711) -> ()  [unwired: 2 in]
                            n686 = case shown="False" w714 {
                              frame #0 {
                                n687 = property on="Load Image" class="Boolean"("Disabled"=u8 0, "Visible"=TRUE) -> ()  [unwired: 2 in, 2 out]
                              }
                              frame #1 {
                                n688 = property on="Load Image" class="Boolean"("Disabled"=u8 2, "Visible"=FALSE) -> ()  [unwired: 2 in, 2 out]
                                n689 = One Button Dialog(message="Die Retrace kann derzeit noch nicht bearbeitet werden.") -> ()  [unwired: 1 in, 1 out]
                              }
                            }
                          }
                          frame #2 {
                            n690 = property on="Image LOADED" class="Boolean (strict)"("Blinking"=TRUE) -> ()  [unwired: 2 in, 2 out]
                            n691 = property on="Image Path" class="Path"("Disabled"=u8 2) -> ()  [unwired: 2 in, 2 out]
                            n692 = property on="Load Image" class="Boolean"("Disabled"=u8 2) -> ()  [unwired: 2 in, 2 out]
                            n693 = call "sumofphotons.vi"("s"=TRUE, "sum of photons"=u32[][][][] []) -> ()  [unwired: 1 out]
                          }
                          frame #3 {
                            n694 = call "TempPath.vi"("change"=FALSE) -> ("stripped path 2"=w735:path)  [unwired: 2 in]
                            n695 = Build Path(base path=w735, name or relative path="Anna_linescan.tmp" ("prompt")) -> (appended path=w733:path)
                            n696 = call <vilib>:"compatOverwrite.vi"("overwrite (F)"=TRUE) -> ("overwrite?"=w728:T13)
                            n697 = Open/Create/Replace Datalog(5:T7 {"router"=[], "macro times"=[], "micro times"=[], "invalid"=[], "gap"=[]} ("cluster"), 10:w728, 11:w733) -> (3:w731:refnum<k1>)  [unwired: 3 in, 2 out]
                            n698 = call "TempRefnum.vi"("change?"=TRUE, "refnum in"=w731) -> ()  [unwired: 1 out]
                          }
                          frame #4 {
                            n699 = property on="LOADED HDR" class="Bool (strict)"() -> ("Value"=w739:bool)  [unwired: 2 in, 2 out]
                            n700 = case shown="True" w739 {
                              frame #0 {
                              }
                              frame #1 {
                                n701 = control-ref of="Image Path"() -> (w741:refnum<vi>)
                                n702 = call "fileformatGlobal.vi"() -> ("fileformat out"=w740:enum16{"Herty", "Ken", "SPC130", "HydraHarp"})  [unwired: 2 in]
                                n703 = case shown="\"SPC130\"" w740 {
                                tunnel: w741 -> [w742 w743 w744]
                                frame #0 {
                                n704 = call "LoadData.vi"("Path"=w742) -> ()  [unwired: 2 in, 3 out]
                                }
                                frame #1 {
                                n705 = call "LoadDataSPC130.vi"("Path"=w743) -> ()  [unwired: 2 in, 3 out]
                                }
                                frame #2 {
                                n706 = call "LoadDataKen.vi"("Path"=w744) -> ()  [unwired: 5 in]
                                }
                                }
                              }
                            }
                          }
                          frame #5 {
                            n707 = call "sumofphotons.vi"("s"=FALSE) -> ("sum of photons out"=w746:u32[][][][])  [unwired: 1 in]
                            n708 = property on="router" class="Ring (strict)"() -> ("Value"=w751:u8)  [unwired: 2 in, 2 out]
                            n709 = property on="plane" class="DigNum (strict)"() -> ("Value"=w750:u32)  [unwired: 2 in, 2 out]
                            n710 = property on="threshold" class="Clust (strict)"() -> ("Value"=w745:cluster{"max":u32, "min":u32})  [unwired: 2 in, 2 out]
                            n711 = property on="RGB or false color?" class="Bool (strict)"() -> ("Value"=w749:bool)  [unwired: 2 in, 2 out]
                            n712 = call "OnlinePic.vi"("action"=T2."ini" ("Enum"), "RGB/False"=w749, "Threshold (max)"=w745, "plane"=w750, "router channel"=w751, "Array"=w746) -> ()  [unwired: 1 in, 5 out]
                          }
                          frame #6 {
                            n713 = call "ViewImageSetnew.vi"("action"=enum16{"Display", "change", "Get", "Set"}."Get" ("Enum")) -> ("Image Settings"=w757:T10)  [unwired: 2 in]
                            n714 = Unbundle By Name(w757) -> ("Image Size (pixel).z"=w756:u32)
                            n715 = case shown="0" w756 {
                              tunnel: [i8 2 w761] -> w755
                              tunnel: [u8 0 w761] -> w754
                              frame #0 {
                              }
                              frame #1 {
                                w761 = u8 0
                              }
                            }
                            n716 = property on="plane" class="DigNum (strict)"("Disabled"=w755, "Value"=w754) -> ()  [unwired: 2 in, 2 out]
                          }
                          frame #7 {
                            w762 = u8 0
                            n717 = property on="Image LOADED" class="Boolean (strict)"("Blinking"=FALSE, "Value"=TRUE ("Image LOADED")) -> ()  [unwired: 2 in, 2 out]
                            n718 = property on="Lifetime pick" class="Boolean"("Disabled"=w762) -> ()  [unwired: 2 in, 2 out]
                            n719 = property on="RGB or false color?" class="Boolean (strict)"("Disabled"=w762) -> ()  [unwired: 2 in, 2 out]
                            n720 = property on="router" class="Ring (strict)"("Disabled"=w762) -> ()  [unwired: 2 in, 2 out]
                            n721 = property on="16bit" class="Boolean"("Disabled"=w762) -> ()  [unwired: 2 in, 2 out]
                            n722 = property on="threshold" class="Clust (strict)"("Disabled"=w762) -> ()  [unwired: 2 in, 2 out]
                            n723 = property on="coincidence spot" class="Boolean"("Disabled"=w762) -> ()  [unwired: 2 in, 2 out]
                            n724 = property on="TAC Window" class="Boolean"("Disabled"=w762) -> ()  [unwired: 2 in, 2 out]
                            n725 = property on="Export" class="Bool"("Disabled"=w762) -> ()  [unwired: 2 in, 2 out]
                            n726 = property on="coincidence\nimage" class="Bool"("Disabled"=w762) -> ()  [unwired: 2 in, 2 out]
                          }
                          frame #8 {
                            n727 = property on="Ampel" class="Clust (strict)"("Value"=cluster{"RED":bool, "RED 2":bool, "RED 3":bool} {"RED"=FALSE, "RED 2"=FALSE, "RED 3"=TRUE} ("Ampel")) -> ()  [unwired: 2 in, 2 out]
                          }
                          frame #9 {
                            n728 = property on="LOADED HDR" class="Boolean (strict)"() -> ("Value"=w767:bool)  [unwired: 2 in, 2 out]
                            n729 = case shown="True" w767 {
                              frame #0 {
                              }
                              frame #1 {
                                w769 = FALSE ("Boolean")
                                w768 = u8 2 ("Disabled")
                                n730 = property on="Image LOADED" class="Boolean (strict)"("Value"=w769, "Blinking"=w769) -> ()  [unwired: 2 in, 2 out]
                                n731 = property on="Spotfinder" class="Boolean"("Disabled"=w768) -> ()  [unwired: 2 in, 2 out]
                                n732 = property on="TAC Window" class="Boolean"("Disabled"=w768) -> ()  [unwired: 2 in, 2 out]
                                n733 = property on="Export" class="Boolean"("Disabled"=w768) -> ()  [unwired: 2 in, 2 out]
                                n734 = property on="View Image Settings" class="Boolean"("Disabled"=w768) -> ()  [unwired: 2 in, 2 out]
                                n735 = property on="View FIFO Settings" class="Boolean"("Disabled"=w768) -> ()  [unwired: 2 in, 2 out]
                              }
                            }
                          }
                          frame #10 {
                            n736 = stacked-sequence {
                              frame #0 {
                                n737 = call "TempRefnum.vi"("change?"=FALSE) -> ("refnum out"=w772:refnum<k1>)  [unwired: 1 in]
                                n738 = Close File(refnum=w772) -> (error out=w770:errorcluster)  [unwired: 1 in, 1 out]
                                n739 = call "HandleError.vi"("error in (no error)"=w770) -> ()
                              }
                              frame #1 {
                                n740 = call "TotalRecall_Reload.vi"() -> ("gap"=w773:i32, "invalid"=w774:i32, "valid"=w775:i32)  [unwired: 4 in, 1 out]
                                n741 = property on="total" class="DigNum (strict)"("Value"=w775) -> ()  [unwired: 2 in, 2 out]
                                n742 = property on="invalid" class="DigNum (strict)"("Value"=w774) -> ()  [unwired: 2 in, 2 out]
                                n743 = property on="gap" class="DigNum (strict)"("Value"=w773) -> ()  [unwired: 2 in, 2 out]
                              }
                            }
                          }
                        }
                      }
                    }
                    frame #1 {
                      n744 = control-ref of="notes"() -> (w776:refnum<vi>)
                      n745 = stacked-sequence {
                        tunnel: w776 -> [w781 w787 _]
                        frame #0 {
                          n746 = property class="Str"(reference=w781) -> (reference out=w780:refnum<vi>, "Value"=w779:string)  [unwired: 1 in, 1 out]
                          n747 = property on="Ampel" class="Clust (strict)"("Value"=cluster{"RED":bool, "YELLOW":bool, "GREEN":bool} {"RED"=FALSE, "YELLOW"=FALSE, "GREEN"=FALSE} ("Ampel")) -> ("Controls[]"=w785:refnum<vi>[])  [unwired: 2 in, 2 out]
                          n748 = Concatenate Strings(w779, "\n- spotfinder\n") -> (w778:string)
                          n749 = Index Array(array=w785, index=1) -> (element=w783:refnum<vi>)
                          n750 = property class="Ctl"(reference=w783, "Blinking"=TRUE) -> ()  [unwired: 1 in, 2 out]
                          n751 = property class="Str"(reference=w780, "Value"=w778) -> ()  [unwired: 1 in, 2 out]
                        }
                        frame #1 {
                          n752 = control-ref of="plane"() -> (w789:refnum<vi>)
                          n753 = control-ref of="TACwinLoaded?"() -> (w791:refnum<vi>)
                          n754 = control-ref of="16btimage?"() -> (w790:refnum<vi>)
                          n755 = control-ref of="router"() -> (w788:refnum<vi>)
                          n756 = control-ref of="Image Path"() -> (w792:refnum<vi>)
                          n757 = control-ref of="Int duplex?"() -> (w793:refnum<vi>)
                          n758 = call "SpotFinder.vi"("Int duplex?"=w793, "notes"=w787, "router 3"=w788, "plane 2"=w789, "Image Path"=w792, "16bit?"=w790, "TACwinLoaded?"=w791) -> ()  [unwired: 4 in]
                        }
                        frame #2 {
                          n759 = property on="Ampel" class="Clust (strict)"("Value"=cluster{"RED":bool, "YELLOW":bool, "GREEN":bool} {"RED"=FALSE, "YELLOW"=FALSE, "GREEN"=TRUE} ("Ampel")) -> ("Controls[]"=w797:refnum<vi>[])  [unwired: 2 in, 2 out]
                          n760 = Index Array(array=w797, index=1) -> (element=w795:refnum<vi>)
                          n761 = property class="Ctl"(reference=w795, "Blinking"=FALSE) -> ()  [unwired: 1 in, 2 out]
                        }
                      }
                    }
                  }
                }
              }
              frame #14 {
                n762 = call "spotfindsettings.vi"("Enum"=T1."load") -> ()  [unwired: 8 in, 3 out]
                n763 = call "StandardSettings.vi"("Enum"=enum16{"Load", "get", "Save", "set"}."Load") -> ("StandardSettings"=w804:T8)  [unwired: 4 in]
                n764 = Unbundle By Name(w804) -> ("threshold"=w800:cluster{"max":u32, "min":u32}, "RGB or false color"=w805:bool)
                n765 = property on="Image LOADED" class="Bool (strict)"() -> ("Value"=w803:bool)  [unwired: 2 in, 2 out]
                n766 = Select(t=u8 0 ("Disabled"), s=w803, f=u8 2) -> (s? t:f=w799:u8)
                n767 = property on="RGB or false color?" class="Boolean (strict)"("Disabled"=w799, "Value"=w805) -> ()  [unwired: 2 in, 2 out]
                n768 = property on="threshold" class="Clust (strict)"("Disabled"=w799, "Value"=w800) -> ()  [unwired: 2 in, 2 out]
              }
              frame #15 {
                n769 = stacked-sequence {
                  frame #0 {
                    n770 = call "StandardSettings.vi"("Enum"=enum16{"Load", "get", "Save", "set"}."Save") -> ()  [unwired: 4 in, 1 out]
                  }
                  frame #1 {
                    n771 = call "spotfindsettings.vi"("Enum"=T1."save") -> ()  [unwired: 8 in, 3 out]
                  }
                }
              }
              frame #16 {
                n772 = control-ref of="notes"() -> (w810:refnum<vi>)
                n773 = call "spotfindsettings.vi"("Enum"=enum16{"Display", "change", "get"}."Display", "notes 2"=w810) -> ()  [unwired: 7 in, 3 out]
              }
              frame #17 {
                n774 = property on="Image Path" class="Path"() -> ("Value"=w812:path)  [unwired: 2 in, 2 out]
                n775 = Not A Number/Path/Refnum?(number/path/refnum=w812) -> (NaN/Path/Refnum?=w813:bool)
                n776 = case shown="False" w813 {
                  tunnel: w812 -> [w821 _]
                  frame #0 {
                    n777 = call "scanSubDir.vi"("path"=w821) -> ("Array"=w819:path[])
                    n778 = call "ScanSubDirGlobal.vi"("set"=TRUE, "Array 2"=w819) -> ()  [unwired: 1 out]
                    n779 = Path To String(path=w819) -> (string=w818:string[])
                    n780 = Array Size(array=w818) -> (size(s)=w817:i32)
                    n781 = Not Equal To 0?(x=w817) -> (x != 0?=w816:bool)
                    n782 = Not(x=w816) -> (.not. x?=w815:bool)
                    n783 = property on="Header Path Ring" class="Ring (strict)"("Strings []"=w818, "Visible"=w816, "Disabled"=u8 0) -> ()  [unwired: 2 in, 2 out]
                    n784 = property on="Image Path" class="Path"("Visible"=w815) -> ()  [unwired: 2 in, 2 out]
                  }
                  frame #1 {
                    n785 = property on="Image Path" class="Path"("Visible"=TRUE) -> ()  [unwired: 2 in, 2 out]
                    n786 = property on="Header Path Ring" class="Ring (strict)"("Visible"=FALSE) -> ()  [unwired: 2 in, 2 out]
                  }
                }
              }
              frame #18 {
                n787 = property on="plane" class="DigNum (strict)"() -> ("Disabled"=w825:u8)  [unwired: 2 in, 2 out]
                n788 = Not Equal To 0?(x=w825) -> (x != 0?=w824:bool)
                n789 = case shown="False" w824 {
                  frame #0 {
                    n790 = call "3dview.vi"() -> ()  [unwired: 7 in]
                  }
                  frame #1 {
                  }
                }
              }
              frame #19 {
                n791 = call "ProfileXY.vi"() -> ()  [unwired: 1 in]
              }
              frame #20 {
                n792 = property on="Image LOADED" class="Boolean (strict)"() -> ("Value"=w826:bool)  [unwired: 2 in, 2 out]
                n793 = case shown="True" w826 {
                  frame #0 {
                  }
                  frame #1 {
                    n794 = call "ConcidenceTesting.vi"() -> ()  [unwired: 1 in]
                  }
                }
              }
            }
          }
          event #17 {
            n795 = event-data() -> ()  [unwired: 1 in, 5 out]
            n796 = property on="LOADED HDR" class="Bool (strict)"() -> ("Value"=w828:bool)  [unwired: 2 in, 2 out]
            n797 = case shown="True" w828 {
              frame #0 {
                n798 = One Button Dialog(message="No data loaded.") -> ()  [unwired: 1 in, 1 out]
              }
              frame #1 {
                n799 = stacked-sequence {
                  frame #0 {
                    n800 = property on="Ampel" class="Clust (strict)"("Value"=cluster{"RED":bool, "RED 2":bool, "RED 3":bool} {"RED"=FALSE, "RED 2"=FALSE, "RED 3"=FALSE} ("Ampel")) -> ()  [unwired: 2 in, 2 out]
                    n801 = property on="YELLOW" class="Boolean (strict)"("Blinking"=TRUE) -> ()  [unwired: 2 in, 2 out]
                  }
                  frame #1 {
                    n802 = case shown="True" "View FIFO Settings" {
                      frame #0 {
                      }
                      frame #1 {
                        n803 = call "ViewFIFOSet.vi"("Enum"=enum16{"Display", "change", "Get", "Set"}."Display") -> ()  [unwired: 1 in, 1 out]
                      }
                    }
                    n804 = case shown="True" "View Image Settings" {
                      frame #0 {
                      }
                      frame #1 {
                        n805 = call "ViewImageSetnew.vi"("action"=enum16{"Display", "change", "Get", "Set"}."Display" ("Enum")) -> ()  [unwired: 2 in, 1 out]
                      }
                    }
                  }
                  frame #2 {
                    n806 = property on="Ampel" class="Clust (strict)"("Value"=cluster{"RED":bool, "RED 2":bool, "RED 3":bool} {"RED"=FALSE, "RED 2"=FALSE, "RED 3"=TRUE} ("Ampel")) -> ()  [unwired: 2 in, 2 out]
                    n807 = property on="YELLOW" class="Boolean (strict)"("Blinking"=FALSE) -> ()  [unwired: 2 in, 2 out]
                  }
                }
              }
            }
          }
          event #18 {
            n808 = event-data() -> ()  [unwired: 1 in, 1 out]
          }
          event #19 {
            n809 = event-data() -> ()  [unwired: 1 in, 3 out]
            n810 = Two Button Dialog(message="Do you really want to quit ANNA_linescan?") -> (T button?=w841:bool)  [unwired: 2 in]
            n811 = Not(x=w841) -> (.not. x?=w840:bool)
            n812 = event-data("Discard?"=w840) -> ()  [unwired: 1 in, 1 out]
          }
        }
      }
    }
    frame #5 {
      n813 = Path To String(path=path "") -> (string=w845:string)
      n814 = Concatenate Strings("Anna_linescan " ("string"), w845) -> (w847:string)
      n815 = call "sumofphotons.vi"("s"=TRUE, "sum of photons"=u32[][][][] []) -> ()  [unwired: 1 out]
      n816 = property class="VI"("Front Panel Window:Title"=w847) -> ()  [unwired: 2 in, 2 out]
      n817 = call "IMAQ GetPalette"() -> ()  [unwired: 5 in, 2 out]
      n818 = call "IMAQ WindClose"("Close All Windows (False)"=TRUE ("Close All Windows (N)")) -> ("error out"=w851:errorcluster)  [unwired: 5 in]
      n819 = property class="VI"("Front Panel Window:Open"=TRUE) -> ()  [unwired: 2 in, 2 out]
      n820 = call "IMAQ WindToolsClose"("error in (no error)"=w851) -> ()  [unwired: 5 in, 1 out]
      n821 = stacked-sequence {
        frame #0 {
          n822 = property on="LOADED HDR" class="Bool (strict)"() -> ("Value"=w853:bool)  [unwired: 2 in, 2 out]
          n823 = case shown="True" w853 {
            frame #0 {
            }
            frame #1 {
              n824 = control-ref of="notes"() -> (w855:refnum<vi>)
              n825 = call "SaveNotes.vi"("Enum"=enum16{"Get Path", "Read", "Save"}."Save", "String"=w855) -> ()  [unwired: 3 in]
            }
          }
        }
        frame #1 {
          n826 = property on="notes" class="String"("Value"="") -> ()  [unwired: 2 in, 2 out]
        }
      }
      n827 = property on="Ampel" class="Clust (strict)"("Value"=cluster{"RED":bool, "RED 2":bool, "RED 3":bool} {"RED"=FALSE, "RED 2"=FALSE, "RED 3"=FALSE} ("Ampel")) -> ()  [unwired: 2 in, 2 out]
      n828 = property on="YELLOW" class="Boolean (strict)"("Blinking"=TRUE) -> ()  [unwired: 2 in, 2 out]
    }
  }
